vi "InitGalvo.vi"(0 "Galvo-resource in":T4, 1 "No of runs (min.)":i32=1, 2 "ScanControl":T5=[{"Time [s]"=0.0, "action"=enum."Abs", "channel"=enum."SMoveTime", "value (/s)"=0.00144}, {"Time [s]"=0.0, "action"=enum."Abs", "channel"=enum."GalvoX", "value (/s)"=-3.625e-05}, {"Time [s]"=0.0, "action"=enum."Abs", "channel"=enum."GalvoY", "value (/s)"=-4.3125e-05}, {"Time [s]"=0.0, "action"=enum."Abs", "channel"=enum."Galvo3", "value (/s)"=0.0}, {"Time [s]"=0.0, "action"=enum."Abs", "channel"=enum."Image1X", "value (/s)"=0.0}, {"Time [s]"=0.0, "action"=enum."Abs", "channel"=enum."Image1Y", "value (/s)"=0.0}, {"Time [s]"=0.0, "action"=enum."Abs", "channel"=enum."AnalogConfig", "value (/s)"=2.0}, {"Time [s]"=0.0, "action"=enum."LoopStart", "channel"=enum."Loop", "value (/s)"=199.0}, {"Time [s]"=0.0, "action"=enum."Inc", "channel"=enum."GalvoX", "value (/s)"=0.0143229167}, {"Time [s]"=0.0, "action"=enum."Inc", "channel"=enum."GalvoY", "value (/s)"=0.0}, {"Time [s]"=0.0, "action"=enum."Inc", "channel"=enum."Galvo3", "value (/s)"=83333.3333333333}, {"Time [s]"=0.0, "action"=enum."Inc", "channel"=enum."Image1X", "value (/s)"=0.0}, {"Time [s]"=1.2e-05, "action"=enum."Inc", "channel"=enum."Image1X", "value (/s)"=83333.3333333333}, {"Time [s]"=0.0048, "action"=enum."Inc", "channel"=enum."Image1X", "value (/s)"=0.0}, {"Time [s]"=0.0048, "action"=enum."Rel", "channel"=enum."Image1Y", "value (/s)"=1.0}, {"Time [s]"=0.004812, "action"=enum."Abs", "channel"=enum."AnalogConfig", "value (/s)"=3.0}, {"Time [s]"=0.004812, "action"=enum."Inc", "channel"=enum."GalvoX", "value (/s)"=3.5717996675e-05}, {"Time [s]"=0.004812, "action"=enum."Inc", "channel"=enum."GalvoY", "value (/s)"=-2.7275561097e-05}, {"Time [s]"=0.004812, "action"=enum."Inc", "channel"=enum."Galvo3", "value (/s)"=0.0}, {"Time [s]"=0.0, "action"=enum."Abs", "channel"=enum."AnalogConfig", "value (/s)"=2.0}, {"Time [s]"=0.0, "action"=enum."Inc", "channel"=enum."GalvoX", "value (/s)"=-0.0143229167}, {"Time [s]"=0.0, "action"=enum."Inc", "channel"=enum."GalvoY", "value (/s)"=0.0}, {"Time [s]"=0.0, "action"=enum."Inc", "channel"=enum."Galvo3", "value (/s)"=-83333.3333333333}, {"Time [s]"=0.0, "action"=enum."Inc", "channel"=enum."Image1X", "value (/s)"=0.0}, {"Time [s]"=1.2e-05, "action"=enum."Inc", "channel"=enum."Image1X", "value (/s)"=-83333.3333333333}, {"Time [s]"=0.0048, "action"=enum."Inc", "channel"=enum."Image1X", "value (/s)"=0.0}, {"Time [s]"=0.0048, "action"=enum."Rel", "channel"=enum."Image1Y", "value (/s)"=1.0}, {"Time [s]"=0.004812, "action"=enum."Abs", "channel"=enum."AnalogConfig", "value (/s)"=3.0}, {"Time [s]"=0.004812, "action"=enum."Inc", "channel"=enum."GalvoX", "value (/s)"=-3.5717996675e-05}, {"Time [s]"=0.004812, "action"=enum."Inc", "channel"=enum."GalvoY", "value (/s)"=-2.7275561097e-05}, {"Time [s]"=0.004812, "action"=enum."Inc", "channel"=enum."Galvo3", "value (/s)"=0.0}, {"Time [s]"=0.0, "action"=enum."Abs", "channel"=enum."AnalogConfig", "value (/s)"=2.0}, {"Time [s]"=0.0, "action"=enum."LoopEnd", "channel"=enum."Loop", "value (/s)"=0.0}, {"Time [s]"=0.0, "action"=enum."Inc", "channel"=enum."GalvoX", "value (/s)"=0.0143229167}, {"Time [s]"=0.0, "action"=enum."Inc", "channel"=enum."GalvoY", "value (/s)"=0.0}, {"Time [s]"=0.0, "action"=enum."Inc", "channel"=enum."Galvo3", "value (/s)"=83333.3333333333}, {"Time [s]"=0.0, "action"=enum."Inc", "channel"=enum."Image1X", "value (/s)"=0.0}, {"Time [s]"=1.2e-05, "action"=enum."Inc", "channel"=enum."Image1X", "value (/s)"=83333.3333333333}, {"Time [s]"=0.0048, "action"=enum."Inc", "channel"=enum."Image1X", "value (/s)"=0.0}, {"Time [s]"=0.0048, "action"=enum."Rel", "channel"=enum."Image1Y", "value (/s)"=1.0}, {"Time [s]"=0.004812, "action"=enum."Abs", "channel"=enum."AnalogConfig", "value (/s)"=3.0}, {"Time [s]"=0.004812, "action"=enum."Inc", "channel"=enum."GalvoX", "value (/s)"=3.5717996675e-05}, {"Time [s]"=0.004812, "action"=enum."Inc", "channel"=enum."GalvoY", "value (/s)"=-2.7275561097e-05}, {"Time [s]"=0.004812, "action"=enum."Inc", "channel"=enum."Galvo3", "value (/s)"=0.0}, {"Time [s]"=0.0, "action"=enum."Abs", "channel"=enum."AnalogConfig", "value (/s)"=2.0}, {"Time [s]"=0.0, "action"=enum."Inc", "channel"=enum."GalvoX", "value (/s)"=-0.0143229167}, {"Time [s]"=0.0, "action"=enum."Inc", "channel"=enum."GalvoY", "value (/s)"=0.0}, {"Time [s]"=0.0, "action"=enum."Inc", "channel"=enum."Galvo3", "value (/s)"=-83333.3333333333}, {"Time [s]"=0.0, "action"=enum."Inc", "channel"=enum."Image1X", "value (/s)"=0.0}, {"Time [s]"=1.2e-05, "action"=enum."Inc", "channel"=enum."Image1X", "value (/s)"=-83333.3333333333}, {"Time [s]"=0.0048, "action"=enum."Inc", "channel"=enum."GalvoX", "value (/s)"=0.0}, {"Time [s]"=0.0048, "action"=enum."Inc", "channel"=enum."GalvoY", "value (/s)"=0.0}, {"Time [s]"=0.0048, "action"=enum."Inc", "channel"=enum."Galvo3", "value (/s)"=0.0}, {"Time [s]"=0.0048, "action"=enum."Inc", "channel"=enum."Image1X", "value (/s)"=0.0}, {"Time [s]"=0.0048, "action"=enum."Abs", "channel"=enum."AnalogConfig", "value (/s)"=0.0}], 3 "Timing":T1={"AD-clock"=4000000.0, "external ADclock"=TRUE, "Galvocycle"=1e-05, "Bitsize"=1e-07, "AD.start.delay"=0.0, "AddStartTriggerIn"=FALSE, "VoltageRange"={"min Voltage"=-0.1, "max Voltage"=10.0}}, 5 "error in (no error)":errorcluster) -> (6 "Galvo-resource out":T4, 7 "Exact duration/run":dbl, 8 "error out":errorcluster={"status"=TRUE, "code"=-1073807339, "source"="VISA Write in InitGalvo.vi->2PhotonImaging_imaq.vi"})   [LabVIEW 2011]
uses:
  Library/ScanControl/ScanControl.ctl
  Library/ScanControl/ScanControl_Action.ctl
  Library/ScanControl/ScanControl_Channel.ctl
  SIAM/SIAM_command.ctl
  SIAM/SIAM-send.ctl
  <vilib>/DAQmx/write.llb/DAQmx Write (Analog 2D I16 NChan NSamp).vi
  <vilib>/DAQmx/create/channels.llb/DAQmx Create Channel (AO-Voltage-Basic).vi
  <vilib>/DAQmx/configure/timing.llb/DAQmx Timing (Sample Clock).vi
  <vilib>/DAQmx/miscellaneous.llb/DAQmx Fill In Error Info.vi
  National Instruments/LabVIEW 2011/resource/objmgr/daqmx.rc
panel:
  out "Tab Control":enum32{"none", "DSP", "Aout", "SIAM"}(tab)=enum."DSP"
  out "Bytes":i32
  out "FromDSP":string
  out "StringToDSP":string="C\nAV,0,3,-663734\r\nAV,0,4,-789615\r\nAV,0,5,0\r\nAI,0,3,3147\r\nAI,0,4,0\r\nAI,0,5,0\r\nAI,0,3,-3147\r\nAI,0,4,0\r\nAI,0,5,0\r\nAI,0,3,3147\r\nAI,0,4,0\r\nAI,0,5,0\r\nAI,0,3,-3147\r\nAI,0,4,0\r\nAI,0,5,0\r\nAI,0,3,3147\r\nAI,0,4,0\r\nAI,0,5,0\r\nAI,0,3,-3147\r\nAI,0,4,0\r\nAI,0,5,0\r\nAI,0,3,3147\r\nAI,0,4,0\r\nAI,0,5,0\r\nAI,0,3,-3147\r\nAI,0,4,0\r\nAI,0,5,0\r\nAI,0,3,3147\r\nAI,0,4,0\r\nAI,0,5,0\r\nAI,0,3,-3147\r\nAI,0,4,0\r\nAI,0,5,0\r\nAI,0,3,3147\r\nAI,0,4,0\r\nAI,0,5,0\r\nAI,0,3,-3147\r\nAI,0,4,0\r\nAI,0,5,0\r\nAI,0,3,3147\r\nAI,0,4,0\r\nAI,0,5,0\r\nAI,0,3,-3147\r\nAI,0,4,0\r\nAI,0,5,0\r\nAI,0,3,3147\r\nAI,0,4,0\r\nAI,0,5,0\r\nAI,0,3,-3147\r\nAI,0,4,0\r\nAI,0,5,0\r\nAI,0,3,3147\r\nAI,0,4,0\r\nAI,0,5,0\r\nAI,0,3,-3147\r\nAI,0,4,0\r\nAI,0,5,0\r\nAI,0,3,3147\r\nAI,0,4,0\r\nAI,0,5,0\r\nAI,0,3,-3147\r\nAI,0,4,0\r\nAI,0,5,0\r\nAI,0,3,3147\r\nAI,0,4,0\r\nAI,0,5,0\r\nAI,0,3,-3147\r\nAI,0,4,0\r\nAI,0,5,0\r\nAI,0,3,3147\r\nAI,0,4,0\r\nAI,0,5,0\r\nAI,0,3,-3147\r\nAI,0,4,0\r\nAI,0,5,0\r\nAI,0,3,3147\r\nAI,0,4,0\r\nAI,0,5,0\r\nAI,0,3,-3147\r\nAI,0,4,0\r\nAI,0,5,0\r\nAI,0,3,3147\r\nAI,0,4,0\r\nAI,0,5,0\r\nAI,0,3,-3147\r\nAI,0,4,0\r\nAI,0,5,0\r\nAI,0,3,3147\r\nAI,0,4,0\r\nAI,0,5,0\r\nAI,0,3,-3147\r\nAI,0,4,0\r\nAI,0,5,0\r\nAI,0,3,3147\r\nAI,0,4,0\r\nAI,0,5,0\r\nAI,0,3,-3147\r\nAI,0,4,0\r\nAI,0,5,0\r\nAI,0,3,3147\r\nAI,0,4,0\r\nAI,0,5,0\r\nAI,0,3,-3147\r\nAI,0,4,0\r\nAI,0,5,0\r\nAI,0,3,3147\r\nAI,0,4,0\r\nAI,0,5,0\r\nAI,0,3,-3147\r\nAI,0,4,0\r\nAI,0,5,0\r\nAI,0,3,3147\r\nAI,0,4,0\r\nAI,0,5,0\r\nAI,0,3,-3147\r\nAI,0,4,0\r\nAI,0,5,0\r\nAI,0,3,3147\r\nAI,0,4,0\r\nAI,0,5,0\r\nAI,0,3,-3147\r\nAI,0,4,0\r\nAI,0,5,0\r\nAI,0,3,3147\r\nAI,0,4,0\r\nAI,0,5,0\r\nAI,0,3,-3147\r\nAI,0,4,0\r\nAI,0,5,0\r\nAI,0,3,3147\r\nAI,0,4,0\r\nAI,0,5,0\r\nAI,0,3,-3147\r\nAI,0,4,0\r\nAI,0,5,0\r\nAI,0,3,3147\r\nAI,0,4,0\r\nAI,0,5,0\r\nAI,0,3,-3147\r\nAI,0,4,0\r\nAI,0,5,0\r\nAI,0,3,3147\r\nAI,0,4,0\r\nAI,0,5,0\r\nAI,0,3,-3147\r\nAI,0,4,0\r\nAI,0,5,0\r\nAI,0,3,3147\r\nAI,0,4,0\r\nAI,0,5,0\r\nAI,0,3,-3147\r\nAI,0,4,0\r\nAI,0,5,0\r\nAI,0,3,3147\r\nAI,0,4,0\r\nAI,0,5,0\r\nAI,0,3,-3147\r\nAI,0,4,0\r\nAI,0,5,0\r\nAI,0,3,3147\r\nAI,0,4,0\r\nAI,0,5,0\r\nAI,0,3,-3147\r\nAI,0,4,0\r\nAI,0,5,0\r\nAI,0,3,3147\r\nAI,0,4,0\r\nAI,0,5,0\r\nAI,0,3,-3147\r\nAI,0,4,0\r\nAI,0,5,0\r\nAI,0,3,3147\r\nAI,0,4,0\r\nAI,0,5,0\r\nAI,0,3,-3147\r\nAI,0,4,0\r\nAI,0,5,0\r\nAI,0,3,3147\r\nAI,0,4,0\r\nAI,0,5,0\r\nAI,0,3,-3147\r\nAI,0,4,0\r\nAI,0,5,0\r\nAI,0,3,3147\r\nAI,0,4,0\r\nAI,0,5,0\r\nAI,0,3,-3147\r\nAI,0,4,0\r\nAI,0,5,0\r\nAI,0,3,3147\r\nAI,0,4,0\r\nAI,0,5,0\r\nAI,0,3,-3147\r\nAI,0,4,0\r\nAI,0,5,0\r\nAI,0,3,3147\r\nAI,0,4,0\r\nAI,0,5,0\r\nAI,0,3,-3147\r\nAI,0,4,0\r\nAI,0,5,0\r\nAI,0,3,3147\r\nAI,0,4,0\r\nAI,0,5,0\r\nAI,0,3,-3147\r\nAI,0,4,0\r\nAI,0,5,0\r\nAI,0,3,3147\r\nAI,0,4,0\r\nAI,0,5,0\r\nAI,0,3,-3147\r\nAI,0,4,0\r\nAI,0,5,0\r\nAI,0,3,3147\r\nAI,0,4,0\r\nAI,0,5,0\r\nAI,0,3,-3147\r\nAI,0,4,0\r\nAI,0,5,0\r\nAI,0,3,3147\r\nAI,0,4,0\r\nAI,0,5,0\r\nAI,0,3,-3147\r\nAI,0,4,0\r\nAI,0,5,0\r\nAI,0,3,3147\r\nAI,0,4,0\r\nAI,0,5,0\r\nAI,0,3,-3147\r\nAI,0,4,0\r\nAI,0,5,0\r\nAI,0,3,3147\r\nAI,0,4,0\r\nAI,0,5,0\r\nAI,0,3,-3147\r\nAI,0,4,0\r\nAI,0,5,0\r\nAI,0,3,3147\r\nAI,0,4,0\r\nAI,0,5,0\r\nAI,0,3,-3147\r\nAI,0,4,0\r\nAI,0,5,0\r\nAI,0,3,3147\r\nAI,0,4,0\r\nAI,0,5,0\r\nAI,0,3,-3147\r\nAI,0,4,0\r\nAI,0,5,0\r\nAI,0,3,3147\r\nAI,0,4,0\r\nAI,0,5,0\r\nAI,0,3,-3147\r\nAI,0,4,0\r\nAI,0,5,0\r\nAI,0,3,3147\r\nAI,0,4,0\r\nAI,0,5,0\r\nAI,0,3,-3147\r\nAI,0,4,0\r\nAI,0,5,0\r\nAI,0,3,3147\r\nAI,0,4,0\r\nAI,0,5,0\r\nAI,0,3,-3147\r\nAI,0,4,0\r\nAI,0,5,0\r\nAI,0,3,3147\r\nAI,0,4,0\r\nAI,0,5,0\r\nAI,0,3,-3147\r\nAI,0,4,0\r\nAI,0,5,0\r\nAI,0,3,3147\r\nAI,0,4,0\r\nAI,0,5,0\r\nAI,0,3,-3147\r\nAI,0,4,0\r\nAI,0,5,0\r\nAI,0,3,3147\r\nAI,0,4,0\r\nAI,0,5,0\r\nAI,0,3,-3147\r\nAI,0,4,0\r\nAI,0,5,0\r\nAI,0,3,3147\r\nAI,0,4,0\r\nAI,0,5,0\r\nAI,0,3,-3147\r\nAI,0,4,0\r\nAI,0,5,0\r\nAI,0,3,3147\r\nAI,0,4,0\r\nAI,0,5,0\r\nAI,0,3,-3147\r\nAI,0,4,0\r\nAI,0,5,0\r\nAI,0,3,3147\r\nAI,0,4,0\r\nAI,0,5,0\r\nAI,0,3,-3147\r\nAI,0,4,0\r\nAI,0,5,0\r\nAI,0,3,3147\r\nAI,0,4,0\r\nAI,0,5,0\r\nAI,0,3,-3147\r\nAI,0,4,0\r\nAI,0,5,0\r\nAI,0,3,3147\r\nAI,0,4,0\r\nAI,0,5,0\r\nAI,0,3,-3147\r\nAI,0,4,0\r\nAI,0,5,0\r\nAI,0,3,3147\r\nAI,0,4,0\r\nAI,0,5,0\r\nAI,0,3,-3147\r\nAI,0,4,0\r\nAI,0,5,0\r\nAI,0,3,3147\r\nAI,0,4,0\r\nAI,0,5,0\r\nAI,0,3,-3147\r\nAI,0,4,0\r\nAI,0,5,0\r\nAI,0,3,3147\r\nAI,0,4,0\r\nAI,0,5,0\r\nAI,0,3,-3147\r\nAI,0,4,0\r\nAI,0,5,0\r\nAI,0,3,3147\r\nAI,0,4,0\r\nAI,0,5,0\r\nAI,0,3,-3147\r\nAI,0,4,0\r\nAI,0,5,0\r\nAI,0,3,3147\r\nAI,0,4,0\r\nAI,0,5,0\r\nAI,0,3,-3147\r\nAI,0,4,0\r\nAI,0,5,0\r\nAI,0,3,3147\r\nAI,0,4,0\r\nAI,0,5,0\r\nAI,0,3,-3147\r\nAI,0,4,0\r\nAI,0,5,0\r\nAI,0,3,3147\r\nAI,0,4,0\r\nAI,0,5,0\r\nAI,0,3,-3147\r\nAI,0,4,0\r\nAI,0,5,0\r\nAI,0,3,3147\r\nAI,0,4,0\r\nAI,0,5,0\r\nAI,0,3,-3147\r\nAI,0,4,0\r\nAI,0,5,0\r\nAI,0,3,3147\r\nAI,0,4,0\r\nAI,0,5,0\r\nAI,0,3,-3147\r\nAI,0,4,0\r\nAI,0,5,0\r\nAI,0,3,3147\r\nAI,0,4,0\r\nAI,0,5,0\r\nAI,0,3,-3147\r\nAI,0,4,0\r\nAI,0,5,0\r\nAI,0,3,3147\r\nAI,0,4,0\r\nAI,0,5,0\r\nAI,0,3,-3147\r\nAI,0,4,0\r\nAI,0,5,0\r\nAI,0,3,3147\r\nAI,0,4,0\r\nAI,0,5,0\r\nAI,0,3,-3147\r\nAI,0,4,0\r\nAI,0,5,0\r\nAI,0,3,3147\r\nAI,0,4,0\r\nAI,0,5,0\r\nAI,0,3,-3147\r\nAI,0,4,0\r\nAI,0,5,0\r\nAI,0,3,3147\r\nAI,0,4,0\r\nAI,0,5,0\r\nAI,0,3,-3147\r\nAI,0,4,0\r\nAI,0,5,0\r\nAI,0,3,3147\r\nAI,0,4,0\r\nAI,0,5,0\r\nAI,0,3,-3147\r\nAI,0,4,0\r\nAI,0,5,0\r\nAI,0,3,3147\r\nAI,0,4,0\r\nAI,0,5,0\r\nAI,0,3,-3147\r\nAI,0,4,0\r\nAI,0,5,0\r\nAI,0,3,3147\r\nAI,0,4,0\r\nAI,0,5,0\r\nAI,0,3,-3147\r\nAI,0,4,0\r\nAI,0,5,0\r\nAI,0,3,3147\r\nAI,0,4,0\r\nAI,0,5,0\r\nAI,0,3,-3147\r\nAI,0,4,0\r\nAI,0,5,0\r\nAI,0,3,3147\r\nAI,0,4,0\r\nAI,0,5,0\r\nAI,0,3,-3147\r\nAI,0,4,0\r\nAI,0,5,0\r\nAI,0,3,3147\r\nAI,0,4,0\r\nAI,0,5,0\r\nAI,0,3,-3147\r\nAI,0,4,0\r\nAI,0,5,0\r\nAI,0,3,3147\r\nAI,0,4,0\r\nAI,0,5,0\r\nAI,0,3,-3147\r\nAI,0,4,0\r\nAI,0,5,0\r\nAI,0,3,3147\r\nAI,0,4,0\r\nAI,0,5,0\r\nAI,0,3,-3147\r\nAI,0,4,0\r\nAI,0,5,0\r\nAI,0,3,3147\r\nAI,0,4,0\r\nAI,0,5,0\r\nAI,0,3,-3147\r\nAI,0,4,0\r\nAI,0,5,0\r\nAI,0,3,3147\r\nAI,0,4,0\r\nAI,0,5,0\r\nAI,0,3,-3147\r\nAI,0,4,0\r\nAI,0,5,0\r\nAI,0,3,3147\r\nAI,0,4,0\r\nAI,0,5,0\r\nAI,0,3,-3147\r\nAI,0,4,0\r\nAI,0,5,0\r\nAI,0,3,3147\r\nAI,0,4,0\r\nAI,0,5,0\r\nAI,0,3,-3147\r\nAI,0,4,0\r\nAI,0,5,0\r\nAI,0,3,3147\r\nAI,0,4,0\r\nAI,0,5,0\r\nAI,0,3,-3147\r\nAI,0,4,0\r\nAI,0,5,0\r\nAI,0,3,3147\r\nAI,0,4,0\r\nAI,0,5,0\r\nAI,0,3,-3147\r\nAI,0,4,0\r\nAI,0,5,0\r\nAI,0,3,3147\r\nAI,0,4,0\r\nAI,0,5,0\r\nAI,0,3,-3147\r\nAI,0,4,0\r\nAI,0,5,0\r\nAI,0,3,3147\r\nAI,0,4,0\r\nAI,0,5,0\r\nAI,0,3,-3147\r\nAI,0,4,0\r\nAI,0,5,0\r\nAI,0,3,3147\r\nAI,0,4,0\r\nAI,0,5,0\r\nAI,0,3,-3147\r\nAI,0,4,0\r\nAI,0,5,0\r\nAI,0,3,3147\r\nAI,0,4,0\r\nAI,0,5,0\r\nAI,0,3,-3147\r\nAI,0,4,0\r\nAI,0,5,0\r\nAI,0,3,3147\r\nAI,0,4,0\r\nAI,0,5,0\r\nAI,0,3,-3147\r\nAI,0,4,0\r\nAI,0,5,0\r\nAI,0,3,3147\r\nAI,0,4,0\r\nAI,0,5,0\r\nAI,0,3,-3147\r\nAI,0,4,0\r\nAI,0,5,0\r\nAI,0,3,3147\r\nAI,0,4,0\r\nAI,0,5,0\r\nAI,0,3,-3147\r\nAI,0,4,0\r\nAI,0,5,0\r\nAI,0,3,3147\r\nAI,0,4,0\r\nAI,0,5,0\r\nAI,0,3,-3147\r\nAI,0,4,0\r\nAI,0,5,0\r\nAI,0,3,3147\r\nAI,0,4,0\r\nAI,0,5,0\r\nAI,0,3,-3147\r\nAI,0,4,0\r\nAI,0,5,0\r\nAI,0,3,3147\r\nAI,0,4,0\r\nAI,0,5,0\r\nAI,0,3,-3147\r\nAI,0,4,0\r\nAI,0,5,0\r\nAI,0,3,3147\r\nAI,0,4,0\r\nAI,0,5,0\r\nAI,0,3,-3147\r\nAI,0,4,0\r\nAI,0,5,0\r\nAI,0,3,3147\r\nAI,0,4,0\r\nAI,0,5,0\r\nAI,0,3,-3147\r\nAI,0,4,0\r\nAI,0,5,0\r\nAI,0,3,3147\r\nAI,0,4,0\r\nAI,0,5,0\r\nAI,0,3,-3147\r\nAI,0,4,0\r\nAI,0,5,0\r\nAI,0,3,3147\r\nAI,0,4,0\r\nAI,0,5,0\r\nAI,0,3,-3147\r\nAI,0,4,0\r\nAI,0,5,0\r\nAI,0,3,3147\r\nAI,0,4,0\r\nAI,0,5,0\r\nAI,0,3,-3147\r\nAI,0,4,0\r\nAI,0,5,0\r\nAI,0,3,3147\r\nAI,0,4,0\r\nAI,0,5,0\r\nAI,0,3,-3147\r\nAI,0,4,0\r\nAI,0,5,0\r\nAI,0,3,3147\r\nAI,0,4,0\r\nAI,0,5,0\r\nAI,0,3,-3147\r\nAI,0,4,0\r\nAI,0,5,0\r\nAI,0,3,3147\r\nAI,0,4,0\r\nAI,0,5,0\r\nAI,0,3,-3147\r\nAI,0,4,0\r\nAI,0,5,0\r\nAI,0,3,3147\r\nAI,0,4,0\r\nAI,0,5,0\r\nAI,0,3,-3147\r\nAI,0,4,0\r\nAI,0,5,0\r\nAI,0,3,3147\r\nAI,0,4,0\r\nAI,0,5,0\r\nAI,0,3,-3147\r\nAI,0,4,0\r\nAI,0,5,0\r\nAI,0,3,3147\r\nAI,0,4,0\r\nAI,0,5,0\r\nAI,0,3,-3147\r\nAI,0,4,0\r\nAI,0,5,0\r\nAI,0,3,3147\r\nAI,0,4,0\r\nAI,0,5,0\r\nAI,0,3,-3147\r\nAI,0,4,0\r\nAI,0,5,0\r\nAI,0,3,3147\r\nAI,0,4,0\r\nAI,0,5,0\r\nAI,0,3,-3147\r\nAI,0,4,0\r\nAI,0,5,0\r\nAI,0,3,3147\r\nAI,0,4,0\r\nAI,0,5,0\r\nAI,0,3,-3147\r\nAI,0,4,0\r\nAI,0,5,0\r\nAI,0,3,3147\r\nAI,0,4,0\r\nAI,0,5,0\r\nAI,0,3,-3147\r\nAI,0,4,0\r\nAI,0,5,0\r\nAI,0,3,3147\r\nAI,0,4,0\r\nAI,0,5,0\r\nAI,0,3,-3147\r\nAI,0,4,0\r\nAI,0,5,0\r\nAI,0,3,3147\r\nAI,0,4,0\r\nAI,0,5,0\r\nAI,0,3,-3147\r\nAI,0,4,0\r\nAI,0,5,0\r\nAI,0,3,3147\r\nAI,0,4,0\r\nAI,0,5,0\r\nAI,0,3,-3147\r\nAI,0,4,0\r\nAI,0,5,0\r\nAI,0,3,3147\r\nAI,0,4,0\r\nAI,0,5,0\r\nAI,0,3,-3147\r\nAI,0,4,0\r\nAI,0,5,0\r\nAI,0,3,3147\r\nAI,0,4,0\r\nAI,0,5,0\r\nAI,0,3,-3147\r\nAI,0,4,0\r\nAI,0,5,0\r\nAI,0,3,3147\r\nAI,0,4,0\r\nAI,0,5,0\r\nAI,0,3,-3147\r\nAI,0,4,0\r\nAI,0,5,0\r\nAI,0,3,3147\r\nAI,0,4,0\r\nAI,0,5,0\r\nAI,0,3,-3147\r\nAI,0,4,0\r\nAI,0,5,0\r\nAI,0,3,3147\r\nAI,0,4,0\r\nAI,0,5,0\r\nAI,0,3,-3147\r\nAI,0,4,0\r\nAI,0,5,0\r\nAI,0,3,3147\r\nAI,0,4,0\r\nAI,0,5,0\r\nAI,0,3,-3147\r\nAI,0,4,0\r\nAI,0,5,0\r\nAI,0,3,3147\r\nAI,0,4,0\r\nAI,0,5,0\r\nAI,0,3,-3147\r\nAI,0,4,0\r\nAI,0,5,0\r\nAI,0,3,3147\r\nAI,0,4,0\r\nAI,0,5,0\r\nAI,0,3,-3147\r\nAI,0,4,0\r\nAI,0,5,0\r\nAI,0,3,3147\r\nAI,0,4,0\r\nAI,0,5,0\r\nAI,0,3,-3147\r\nAI,0,4,0\r\nAI,0,5,0\r\nAI,0,3,3147\r\nAI,0,4,0\r\nAI,0,5,0\r\nAI,0,3,-3147\r\nAI,0,4,0\r\nAI,0,5,0\r\nAI,0,3,3147\r\nAI,0,4,0\r\nAI,0,5,0\r\nAI,0,3,-3147\r\nAI,0,4,0\r\nAI,0,5,0\r\nAI,0,3,3147\r\nAI,0,4,0\r\nAI,0,5,0\r\nAI,0,3,-3147\r\nAI,0,4,0\r\nAI,0,5,0\r\nAI,0,3,3147\r\nAI,0,4,0\r\nAI,0,5,0\r\nAI,0,3,-3147\r\nAI,0,4,0\r\nAI,0,5,0\r\nAI,0,3,3147\r\nAI,0,4,0\r\nAI,0,5,0\r\nAI,0,3,-3147\r\nAI,0,4,0\r\nAI,0,5,0\r\nAI,0,3,3147\r\nAI,0,4,0\r\nAI,0,5,0\r\nAI,0,3,-3147\r\nAI,0,4,0\r\nAI,0,5,0\r\nAI,0,3,3147\r\nAI,0,4,0\r\nAI,0,5,0\r\nAI,0,3,-3147\r\nAI,0,4,0\r\nAI,0,5,0\r\nAI,0,3,3147\r\nAI,0,4,0\r\nAI,0,5,0\r\nAI,0,3,-3147\r\nAI,0,4,0\r\nAI,0,5,0\r\nAI,0,3,3147\r\nAI,0,4,0\r\nAI,0,5,0\r\nAI,0,3,-3147\r\nAI,0,4,0\r\nAI,0,5,0\r\nAI,0,3,3147\r\nAI,0,4,0\r\nAI,0,5,0\r\nAI,0,3,-3147\r\nAI,0,4,0\r\nAI,0,5,0\r\nAI,0,3,3147\r\nAI,0,4,0\r\nAI,0,5,0\r\nAI,0,3,-3147\r\nAI,0,4,0\r\nAI,0,5,0\r\nAI,0,3,3147\r\nAI,0,4,0\r\nAI,0,5,0\r\nAI,0,3,-3147\r\nAI,0,4,0\r\nAI,0,5,0\r\nAI,0,3,3147\r\nAI,0,4,0\r\nAI,0,5,0\r\nAI,0,3,-3147\r\nAI,0,4,0\r\nAI,0,5,0\r\nAI,0,3,3147\r\nAI,0,4,0\r\nAI,0,5,0\r\nAI,0,3,-3147\r\nAI,0,4,0\r\nAI,0,5,0\r\nAI,0,3,3147\r\nAI,0,4,0\r\nAI,0,5,0\r\nAI,0,3,-3147\r\nAI,0,4,0\r\nAI,0,5,0\r\nAI,0,3,3147\r\nAI,0,4,0\r\nAI,0,5,0\r\nAI,0,3,-3147\r\nAI,0,4,0\r\nAI,0,5,0\r\nAI,0,3,3147\r\nAI,0,4,0\r\nAI,0,5,0\r\nAI,0,3,-3147\r\nAI,0,4,0\r\nAI,0,5,0\r\nAI,0,3,3147\r\nAI,0,4,0\r\nAI,0,5,0\r\nAI,0,3,-3147\r\nAI,0,4,0\r\nAI,0,5,0\r\nAI,0,3,3147\r\nAI,0,4,0\r\nAI,0,5,0\r\nAI,0,3,-3147\r\nAI,0,4,0\r\nAI,0,5,0\r\nAI,0,3,3147\r\nAI,0,4,0\r\nAI,0,5,0\r\nAI,0,3,-3147\r\nAI,0,4,0\r\nAI,0,5,0\r\nAI,0,3,3147\r\nAI,0,4,0\r\nAI,0,5,0\r\nAI,0,3,-3147\r\nAI,0,4,0\r\nAI,0,5,0\r\nAI,0,3,3147\r\nAI,0,4,0\r\nAI,0,5,0\r\nAI,0,3,-3147\r\nAI,0,4,0\r\nAI,0,5,0\r\nAI,0,3,3147\r\nAI,0,4,0\r\nAI,0,5,0\r\nAI,0,3,-3147\r\nAI,0,4,0\r\nAI,0,5,0\r\nAI,0,3,3147\r\nAI,0,4,0\r\nAI,0,5,0\r\nAI,0,3,-3147\r\nAI,0,4,0\r\nAI,0,5,0\r\nAI,0,3,3147\r\nAI,0,4,0\r\nAI,0,5,0\r\nAI,0,3,-3147\r\nAI,0,4,0\r\nAI,0,5,0\r\nAI,0,3,3147\r\nAI,0,4,0\r\nAI,0,5,0\r\nAI,0,3,-3147\r\nAI,0,4,0\r\nAI,0,5,0\r\nAI,0,3,3147\r\nAI,0,4,0\r\nAI,0,5,0\r\nAI,0,3,-3147\r\nAI,0,4,0\r\nAI,0,5,0\r\nAI,0,3,3147\r\nAI,0,4,0\r\nAI,0,5,0\r\nAI,0,3,-3147\r\nAI,0,4,0\r\nAI,0,5,0\r\nAI,0,3,3147\r\nAI,0,4,0\r\nAI,0,5,0\r\nAI,0,3,-3147\r\nAI,0,4,0\r\nAI,0,5,0\r\nAI,0,3,3147\r\nAI,0,4,0\r\nAI,0,5,0\r\nAI,0,3,-3147\r\nAI,0,4,0\r\nAI,0,5,0\r\nAI,0,3,3147\r\nAI,0,4,0\r\nAI,0,5,0\r\nAI,0,3,-3147\r\nAI,0,4,0\r\nAI,0,5,0\r\nAI,0,3,3147\r\nAI,0,4,0\r\nAI,0,5,0\r\nAI,0,3,-3147\r\nAI,0,4,0\r\nAI,0,5,0\r\nAI,0,3,3147\r\nAI,0,4,0\r\nAI,0,5,0\r\nAI,0,3,-3147\r\nAI,0,4,0\r\nAI,0,5,0\r\nAI,0,3,3147\r\nAI,0,4,0\r\nAI,0,5,0\r\nAI,0,3,-3147\r\nAI,0,4,0\r\nAI,0,5,0\r\nAI,0,3,3147\r\nAI,0,4,0\r\nAI,0,5,0\r\nAI,0,3,-3147\r\nAI,0,4,0\r\nAI,0,5,0\r\nAI,0,3,3147\r\nAI,0,4,0\r\nAI,0,5,0\r\nAI,0,3,-3147\r\nAI,0,4,0\r\nAI,0,5,0\r\nAI,0,3,3147\r\nAI,0,4,0\r\nAI,0,5,0\r\nAI,0,3,-3147\r\nAI,0,4,0\r\nAI,0,5,0\r\nAI,0,3,3147\r\nAI,0,4,0\r\nAI,0,5,0\r\nAI,0,3,-3147\r\nAI,0,4,0\r\nAI,0,5,0\r\nAI,0,3,3147\r\nAI,0,4,0\r\nAI,0,5,0\r\nAI,0,3,-3147\r\nAI,0,4,0\r\nAI,0,5,0\r\nAI,0,3,3147\r\nAI,0,4,0\r\nAI,0,5,0\r\nAI,0,3,-3147\r\nAI,0,4,0\r\nAI,0,5,0\r\nAI,0,3,3147\r\nAI,0,4,0\r\nAI,0,5,0\r\nAI,0,3,-3147\r\nAI,0,4,0\r\nAI,0,5,0\r\nAI,0,3,3147\r\nAI,0,4,0\r\nAI,0,5,0\r\nAI,0,3,-3147\r\nAI,0,4,0\r\nAI,0,5,0\r\nAI,0,3,3147\r\nAI,0,4,0\r\nAI,0,5,0\r\nAI,0,3,-3147\r\nAI,0,4,0\r\nAI,0,5,0\r\nAI,0,3,3147\r\nAI,0,4,0\r\nAI,0,5,0\r\nAI,0,3,-3147\r\nAI,0,4,0\r\nAI,0,5,0\r\nAI,0,3,3147\r\nAI,0,4,0\r\nAI,0,5,0\r\nAI,0,3,-3147\r\nAI,0,4,0\r\nAI,0,5,0\r\nAI,0,3,3147\r\nAI,0,4,0\r\nAI,0,5,0\r\nAI,0,3,-3147\r\nAI,0,4,0\r\nAI,0,5,0\r\nAI,0,3,3147\r\nAI,0,4,0\r\nAI,0,5,0\r\nAI,0,3,-3147\r\nAI,0,4,0\r\nAI,0,5,0\r\nAI,0,3,3147\r\nAI,0,4,0\r\nAI,0,5,0\r\nAI,0,3,-3147\r\nAI,0,4,0\r\nAI,0,5,0\r\nAI,0,3,3147\r\nAI,0,4,0\r\nAI,0,5,0\r\nAI,0,3,-3147\r\nAI,0,4,0\r\nAI,0,5,0\r\nAI,0,3,3147\r\nAI,0,4,0\r\nAI,0,5,0\r\nAI,0,3,-3147\r\nAI,0,4,0\r\nAI,0,5,0\r\nAI,0,3,3147\r\nAI,0,4,0\r\nAI,0,5,0\r\nAI,0,3,-3147\r\nAI,0,4,0\r\nAI,0,5,0\r\nAI,0,3,3147\r\nAI,0,4,0\r\nAI,0,5,0\r\nAI,0,3,-3147\r\nAI,0,4,0\r\nAI,0,5,0\r\nAI,0,3,3147\r\nAI,0,4,0\r\nAI,0,5,0\r\nAI,0,3,-3147\r\nAI,0,4,0\r\nAI,0,5,0\r\nAI,0,3,3147\r\nAI,0,4,0\r\nAI,0,5,0\r\nAI,0,3,-3147\r\nAI,0,4,0\r\nAI,0,5,0\r\nAI,0,3,3147\r\nAI,0,4,0\r\nAI,0,5,0\r\nAI,0,3,-3147\r\nAI,0,4,0\r\nAI,0,5,0\r\nAI,0,3,3147\r\nAI,0,4,0\r\nAI,0,5,0\r\nAI,0,3,-3147\r\nAI,0,4,0\r\nAI,0,5,0\r\nAI,0,3,3147\r\nAI,0,4,0\r\nAI,0,5,0\r\nAI,0,3,-3147\r\nAI,0,4,0\r\nAI,0,5,0\r\nAI,0,3,3147\r\nAI,0,4,0\r\nAI,0,5,0\r\nAI,0,3,-3147\r\nAI,0,4,0\r\nAI,0,5,0\r\nAI,0,3,3147\r\nAI,0,4,0\r\nAI,0,5,0\r\nAI,0,3,-3147\r\nAI,0,4,0\r\nAI,0,5,0\r\nAI,0,3,3147\r\nAI,0,4,0\r\nAI,0,5,0\r\nAI,0,3,-3147\r\nAI,0,4,0\r\nAI,0,5,0\r\nAI,0,3,3147\r\nAI,0,4,0\r\nAI,0,5,0\r\nAI,0,3,-3147\r\nAI,0,4,0\r\nAI,0,5,0\r\nAI,0,3,3147\r\nAI,0,4,0\r\nAI,0,5,0\r\nAI,0,3,-3147\r\nAI,0,4,0\r\nAI,0,5,0\r\nAI,0,3,3147\r\nAI,0,4,0\r\nAI,0,5,0\r\nAI,0,3,-3147\r\nAI,0,4,0\r\nAI,0,5,0\r\nAI,0,3,3147\r\nAI,0,4,0\r\nAI,0,5,0\r\nAI,0,3,-3147\r\nAI,0,4,0\r\nAI,0,5,0\r\nAI,0,3,3147\r\nAI,0,4,0\r\nAI,0,5,0\r\nAI,0,3,-3147\r\nAI,0,4,0\r\nAI,0,5,0\r\nAI,0,3,3147\r\nAI,0,4,0\r\nAI,0,5,0\r\nAI,0,3,-3147\r\nAI,0,4,0\r\nAI,0,5,0\r\nAI,0,3,3147\r\nAI,0,4,0\r\nAI,0,5,0\r\nAI,0,3,-3147\r\nAI,0,4,0\r\nAI,0,5,0\r\nAI,0,3,3147\r\nAI,0,4,0\r\nAI,0,5,0\r\nAI,0,3,-3147\r\nAI,0,4,0\r\nAI,0,5,0\r\nAI,0,3,3147\r\nAI,0,4,0\r\nAI,0,5,0\r\nAI,0,3,-3147\r\nAI,0,4,0\r\nAI,0,5,0\r\nAI,0,3,3147\r\nAI,0,4,0\r\nAI,0,5,0\r\nAI,0,3,-3147\r\nAI,0,4,0\r\nAI,0,5,0\r\nAI,0,3,3147\r\nAI,0,4,0\r\nAI,0,5,0\r\nAI,0,3,-3147\r\nAI,0,4,0\r\nAI,0,5,0\r\nAI,0,3,3147\r\nAI,0,4,0\r\nAI,0,5,0\r\nAI,0,3,-3147\r\nAI,0,4,0\r\nAI,0,5,0\r\nAI,0,3,3147\r\nAI,0,4,0\r\nAI,0,5,0\r\nAI,0,3,-3147\r\nAI,0,4,0\r\nAI,0,5,0\r\nAI,0,3,3147\r\nAI,0,4,0\r\nAI,0,5,0\r\nAI,0,3,-3147\r\nAI,0,4,0\r\nAI,0,5,0\r\nAI,0,3,3147\r\nAI,0,4,0\r\nAI,0,5,0\r\nAI,0,3,-3147\r\nAI,0,4,0\r\nAI,0,5,0\r\nAI,0,3,3147\r\nAI,0,4,0\r\nAI,0,5,0\r\nAI,0,3,-3147\r\nAI,0,4,0\r\nAI,0,5,0\r\nAI,0,3,3147\r\nAI,0,4,0\r\nAI,0,5,0\r\nAI,0,3,-3147\r\nAI,0,4,0\r\nAI,0,5,0\r\nAI,0,3,3147\r\nAI,0,4,0\r\nAI,0,5,0\r\nAI,0,3,-3147\r\nAI,0,4,0\r\nAI,0,5,0\r\nAI,0,3,3147\r\nAI,0,4,0\r\nAI,0,5,0\r\nAI,0,3,-3147\r\nAI,0,4,0\r\nAI,0,5,0\r\nAI,0,3,3147\r\nAI,0,4,0\r\nAI,0,5,0\r\nAI,0,3,-3147\r\nAI,0,4,0\r\nAI,0,5,0\r\nAI,0,3,3147\r\nAI,0,4,0\r\nAI,0,5,0\r\nAI,0,3,-3147\r\nAI,0,4,0\r\nAI,0,5,0\r\nAI,0,3,3147\r\nAI,0,4,0\r\nAI,0,5,0\r\nAI,0,3,-3147\r\nAI,0,4,0\r\nAI,0,5,0\r\nAI,0,3,3147\r\nAI,0,4,0\r\nAI,0,5,0\r\nAI,0,3,-3147\r\nAI,0,4,0\r\nAI,0,5,0\r\nAV,120,1,2\r\nAV,120,1,2\r\nAV,120,1,2\r\nAV,120,1,2\r\nAV,120,1,2\r\nAV,120,1,2\r\nAV,120,1,2\r\nAV,120,1,2\r\nAV,120,1,2\r\nAV,120,1,2\r\nAV,120,1,2\r\nAV,120,1,2\r\nAV,120,1,2\r\nAV,120,1,2\r\nAV,120,1,2\r\nAV,120,1,2\r\nAV,120,1,2\r\nAV,120,1,2\r\nAV,120,1,2\r\nAV,120,1,2\r\nAV,120,1,2\r\nAV,120,1,2\r\nAV,120,1,2\r\nAV,120,1,2\r\nAV,120,1,2\r\nAV,120,1,2\r\nAV,120,1,2\r\nAV,120,1,2\r\nAV,120,1,2\r\nAV,120,1,2\r\nAV,120,1,2\r\nAV,120,1,2\r\nAV,120,1,2\r\nAV,120,1,2\r\nAV,120,1,2\r\nAV,120,1,2\r\nAV,120,1,2\r\nAV,120,1,2\r\nAV,120,1,2\r\nAV,120,1,2\r\nAV,120,1,2\r\nAV,120,1,2\r\nAV,120,1,2\r\nAV,120,1,2\r\nAV,120,1,2\r\nAV,120,1,2\r\nAV,120,1,2\r\nAV,120,1,2\r\nAV,120,1,2\r\nAV,120,1,2\r\nAV,120,1,2\r\nAV,120,1,2\r\nAV,120,1,2\r\nAV,120,1,2\r\nAV,120,1,2\r\nAV,120,1,2\r\nAV,120,1,2\r\nAV,120,1,2\r\nAV,120,1,2\r\nAV,120,1,2\r\nAV,120,1,2\r\nAV,120,1,2\r\nAV,120,1,2\r\nAV,120,1,2\r\nAV,120,1,2\r\nAV,120,1,2\r\nAV,120,1,2\r\nAV,120,1,2\r\nAV,120,1,2\r\nAV,120,1,2\r\nAV,120,1,2\r\nAV,120,1,2\r\nAV,120,1,2\r\nAV,120,1,2\r\nAV,120,1,2\r\nAV,120,1,2\r\nAV,120,1,2\r\nAV,120,1,2\r\nAV,120,1,2\r\nAV,120,1,2\r\nAV,120,1,2\r\nAV,120,1,2\r\nAV,120,1,2\r\nAV,120,1,2\r\nAV,120,1,2\r\nAV,120,1,2\r\nAV,120,1,2\r\nAV,120,1,2\r\nAV,120,1,2\r\nAV,120,1,2\r\nAV,120,1,2\r\nAV,120,1,2\r\nAV,120,1,2\r\nAV,120,1,2\r\nAV,120,1,2\r\nAV,120,1,2\r\nAV,120,1,2\r\nAV,120,1,2\r\nAV,120,1,2\r\nAV,120,1,2\r\nAV,120,1,2\r\nAV,120,1,2\r\nAV,120,1,2\r\nAV,120,1,2\r\nAV,120,1,2\r\nAV,120,1,2\r\nAV,120,1,2\r\nAV,120,1,2\r\nAV,120,1,2\r\nAV,120,1,2\r\nAV,120,1,2\r\nAV,120,1,2\r\nAV,120,1,2\r\nAV,120,1,2\r\nAV,120,1,2\r\nAV,120,1,2\r\nAV,120,1,2\r\nAV,120,1,2\r\nAV,120,1,2\r\nAV,120,1,2\r\nAV,120,1,2\r\nAV,120,1,2\r\nAV,120,1,2\r\nAV,120,1,2\r\nAV,120,1,2\r\nAV,120,1,2\r\nAV,120,1,2\r\nAV,120,1,2\r\nAV,120,1,2\r\nAV,120,1,2\r\nAV,120,1,2\r\nAV,120,1,2\r\nAV,120,1,2\r\nAV,120,1,2\r\nAV,120,1,2\r\nAV,120,1,2\r\nAV,120,1,2\r\nAV,120,1,2\r\nAV,120,1,2\r\nAV,120,1,2\r\nAV,120,1,2\r\nAV,120,1,2\r\nAV,120,1,2\r\nAV,120,1,2\r\nAV,120,1,2\r\nAV,120,1,2\r\nAV,120,1,2\r\nAV,120,1,2\r\nAV,120,1,2\r\nAV,120,1,2\r\nAV,120,1,2\r\nAV,120,1,2\r\nAV,120,1,2\r\nAV,120,1,2\r\nAV,120,1,2\r\nAV,120,1,2\r\nAV,120,1,2\r\nAV,120,1,2\r\nAV,120,1,2\r\nAV,120,1,2\r\nAV,120,1,2\r\nAV,120,1,2\r\nAV,120,1,2\r\nAV,120,1,2\r\nAV,120,1,2\r\nAV,120,1,2\r\nAV,120,1,2\r\nAV,120,1,2\r\nAV,120,1,2\r\nAV,120,1,2\r\nAV,120,1,2\r\nAV,120,1,2\r\nAV,120,1,2\r\nAV,120,1,2\r\nAV,120,1,2\r\nAV,120,1,2\r\nAV,120,1,2\r\nAV,120,1,2\r\nAV,120,1,2\r\nAV,120,1,2\r\nAV,120,1,2\r\nAV,120,1,2\r\nAV,120,1,2\r\nAV,120,1,2\r\nAV,120,1,2\r\nAV,120,1,2\r\nAV,120,1,2\r\nAV,120,1,2\r\nAV,120,1,2\r\nAV,120,1,2\r\nAV,120,1,2\r\nAV,120,1,2\r\nAV,120,1,2\r\nAV,120,1,2\r\nAV,120,1,2\r\nAV,120,1,2\r\nAV,120,1,2\r\nAV,120,1,2\r\nAV,120,1,2\r\nAV,120,1,2\r\nAV,120,1,2\r\nAV,120,1,2\r\nAV,120,1,2\r\nAV,120,1,2\r\nAV,120,1,2\r\nAV,120,1,2\r\nAV,120,1,2\r\nAV,120,1,2\r\nAV,120,1,2\r\nAV,120,1,2\r\nAV,120,1,2\r\nAV,120,1,2\r\nAV,120,1,2\r\nAV,120,1,2\r\nAV,120,1,2\r\nAV,120,1,2\r\nAV,120,1,2\r\nAV,120,1,2\r\nAV,120,1,2\r\nAV,120,1,2\r\nAV,120,1,2\r\nAV,120,1,2\r\nAV,120,1,2\r\nAV,120,1,2\r\nAV,120,1,2\r\nAV,120,1,2\r\nAV,120,1,2\r\nAV,120,1,2\r\nAV,120,1,2\r\nAV,120,1,2\r\nAV,120,1,2\r\nAV,120,1,2\r\nAV,120,1,2\r\nAV,120,1,2\r\nAV,120,1,2\r\nAV,120,1,2\r\nAV,120,1,2\r\nAV,120,1,2\r\nAV,120,1,2\r\nAV,120,1,2\r\nAV,120,1,2\r\nAV,120,1,2\r\nAV,120,1,2\r\nAV,120,1,2\r\nAV,120,1,2\r\nAV,120,1,2\r\nAV,120,1,2\r\nAV,120,1,2\r\nAV,120,1,2\r\nAV,120,1,2\r\nAV,120,1,2\r\nAV,120,1,2\r\nAV,120,1,2\r\nAV,120,1,2\r\nAV,120,1,2\r\nAV,120,1,2\r\nAV,120,1,2\r\nAV,120,1,2\r\nAV,120,1,2\r\nAV,120,1,2\r\nAV,120,1,2\r\nAV,120,1,2\r\nAV,120,1,2\r\nAV,120,1,2\r\nAV,120,1,2\r\nAV,120,1,2\r\nAV,120,1,2\r\nAV,120,1,2\r\nAV,120,1,2\r\nAV,120,1,2\r\nAV,120,1,2\r\nAV,120,1,2\r\nAV,120,1,2\r\nAV,120,1,2\r\nAV,120,1,2\r\nAV,120,1,2\r\nAV,120,1,2\r\nAV,120,1,2\r\nAV,120,1,2\r\nAV,120,1,2\r\nAV,120,1,2\r\nAV,120,1,2\r\nAV,120,1,2\r\nAV,120,1,2\r\nAV,120,1,2\r\nAV,120,1,2\r\nAV,120,1,2\r\nAV,120,1,2\r\nAV,120,1,2\r\nAV,120,1,2\r\nAV,120,1,2\r\nAV,120,1,2\r\nAV,120,1,2\r\nAV,120,1,2\r\nAV,120,1,2\r\nAV,120,1,2\r\nAV,120,1,2\r\nAV,120,1,2\r\nAV,120,1,2\r\nAV,120,1,2\r\nAV,120,1,2\r\nAV,120,1,2\r\nAV,120,1,2\r\nAV,120,1,2\r\nAV,120,1,2\r\nAV,120,1,2\r\nAV,120,1,2\r\nAV,120,1,2\r\nAV,120,1,2\r\nAV,120,1,2\r\nAV,120,1,2\r\nAV,120,1,2\r\nAV,120,1,2\r\nAV,120,1,2\r\nAV,120,1,2\r\nAV,120,1,2\r\nAV,120,1,2\r\nAV,120,1,2\r\nAV,120,1,2\r\nAV,120,1,2\r\nAV,120,1,2\r\nAV,120,1,2\r\nAV,120,1,2\r\nAV,120,1,2\r\nAV,120,1,2\r\nAV,120,1,2\r\nAV,120,1,2\r\nAV,120,1,2\r\nAV,120,1,2\r\nAV,120,1,2\r\nAV,120,1,2\r\nAV,120,1,2\r\nAV,120,1,2\r\nAV,120,1,2\r\nAV,120,1,2\r\nAV,120,1,2\r\nAV,120,1,2\r\nAV,120,1,2\r\nAV,120,1,2\r\nAV,120,1,2\r\nAV,120,1,2\r\nAV,120,1,2\r\nAV,120,1,2\r\nAV,120,1,2\r\nAV,120,1,2\r\nAV,120,1,2\r\nAV,120,1,2\r\nAV,120,1,2\r\nAV,120,1,2\r\nAV,120,1,2\r\nAV,120,1,2\r\nAV,120,1,2\r\nAV,120,1,2\r\nAV,120,1,2\r\nAV,120,1,2\r\nAV,120,1,2\r\nAV,120,1,2\r\nAV,120,1,2\r\nAV,120,1,2\r\nAV,120,1,2\r\nAV,120,1,2\r\nAV,120,1,2\r\nAV,120,1,2\r\nAV,120,1,2\r\nAV,120,1,2\r\nAV,120,1,2\r\nAV,120,1,2\r\nAV,120,1,2\r\nAV,120,1,2\r\nAV,120,1,2\r\nAV,120,1,2\r\nAV,120,1,2\r\nAV,120,1,2\r\nAV,120,1,2\r\nAV,120,1,2\r\nAV,120,1,2\r\nAV,120,1,2\r\nAV,120,1,2\r\nAV,120,1,2\r\nAV,120,1,2\r\nAV,120,1,2\r\nAV,120,1,2\r\nAV,120,1,2\r\nAV,120,1,2\r\nAV,120,1,2\r\nAV,120,1,2\r\nAV,120,1,2\r\nAV,120,1,2\r\nAV,120,1,2\r\nAV,120,1,2\r\nAV,120,1,2\r\nAV,120,1,2\r\nAV,120,1,2\r\nAV,120,1,2\r\nAV,120,1,2\r\nAV,120,1,2\r\nAV,120,1,2\r\nAV,120,1,2\r\nAV,120,1,2\r\nAV,120,1,2\r\nAI,400,3,0\r\nAI,400,4,0\r\nAI,400,5,0\r\nAI,401,3,8\r\nAI,401,4,-6\r\nAI,401,5,0\r\nAI,401,3,-8\r\nAI,401,4,-6\r\nAI,401,5,0\r\nAI,401,3,8\r\nAI,401,4,-6\r\nAI,401,5,0\r\nAI,401,3,-8\r\nAI,401,4,-6\r\nAI,401,5,0\r\nAI,401,3,8\r\nAI,401,4,-6\r\nAI,401,5,0\r\nAI,401,3,-8\r\nAI,401,4,-6\r\nAI,401,5,0\r\nAI,401,3,8\r\nAI,401,4,-6\r\nAI,401,5,0\r\nAI,401,3,-8\r\nAI,401,4,-6\r\nAI,401,5,0\r\nAI,401,3,8\r\nAI,401,4,-6\r\nAI,401,5,0\r\nAI,401,3,-8\r\nAI,401,4,-6\r\nAI,401,5,0\r\nAI,401,3,8\r\nAI,401,4,-6\r\nAI,401,5,0\r\nAI,401,3,-8\r\nAI,401,4,-6\r\nAI,401,5,0\r\nAI,401,3,8\r\nAI,401,4,-6\r\nAI,401,5,0\r\nAI,401,3,-8\r\nAI,401,4,-6\r\nAI,401,5,0\r\nAI,401,3,8\r\nAI,401,4,-6\r\nAI,401,5,0\r\nAI,401,3,-8\r\nAI,401,4,-6\r\nAI,401,5,0\r\nAI,401,3,8\r\nAI,401,4,-6\r\nAI,401,5,0\r\nAI,401,3,-8\r\nAI,401,4,-6\r\nAI,401,5,0\r\nAI,401,3,8\r\nAI,401,4,-6\r\nAI,401,5,0\r\nAI,401,3,-8\r\nAI,401,4,-6\r\nAI,401,5,0\r\nAI,401,3,8\r\nAI,401,4,-6\r\nAI,401,5,0\r\nAI,401,3,-8\r\nAI,401,4,-6\r\nAI,401,5,0\r\nAI,401,3,8\r\nAI,401,4,-6\r\nAI,401,5,0\r\nAI,401,3,-8\r\nAI,401,4,-6\r\nAI,401,5,0\r\nAI,401,3,8\r\nAI,401,4,-6\r\nAI,401,5,0\r\nAI,401,3,-8\r\nAI,401,4,-6\r\nAI,401,5,0\r\nAI,401,3,8\r\nAI,401,4,-6\r\nAI,401,5,0\r\nAI,401,3,-8\r\nAI,401,4,-6\r\nAI,401,5,0\r\nAI,401,3,8\r\nAI,401,4,-6\r\nAI,401,5,0\r\nAI,401,3,-8\r\nAI,401,4,-6\r\nAI,401,5,0\r\nAI,401,3,8\r\nAI,401,4,-6\r\nAI,401,5,0\r\nAI,401,3,-8\r\nAI,401,4,-6\r\nAI,401,5,0\r\nAI,401,3,8\r\nAI,401,4,-6\r\nAI,401,5,0\r\nAI,401,3,-8\r\nAI,401,4,-6\r\nAI,401,5,0\r\nAI,401,3,8\r\nAI,401,4,-6\r\nAI,401,5,0\r\nAI,401,3,-8\r\nAI,401,4,-6\r\nAI,401,5,0\r\nAI,401,3,8\r\nAI,401,4,-6\r\nAI,401,5,0\r\nAI,401,3,-8\r\nAI,401,4,-6\r\nAI,401,5,0\r\nAI,401,3,8\r\nAI,401,4,-6\r\nAI,401,5,0\r\nAI,401,3,-8\r\nAI,401,4,-6\r\nAI,401,5,0\r\nAI,401,3,8\r\nAI,401,4,-6\r\nAI,401,5,0\r\nAI,401,3,-8\r\nAI,401,4,-6\r\nAI,401,5,0\r\nAI,401,3,8\r\nAI,401,4,-6\r\nAI,401,5,0\r\nAI,401,3,-8\r\nAI,401,4,-6\r\nAI,401,5,0\r\nAI,401,3,8\r\nAI,401,4,-6\r\nAI,401,5,0\r\nAI,401,3,-8\r\nAI,401,4,-6\r\nAI,401,5,0\r\nAI,401,3,8\r\nAI,401,4,-6\r\nAI,401,5,0\r\nAI,401,3,-8\r\nAI,401,4,-6\r\nAI,401,5,0\r\nAI,401,3,8\r\nAI,401,4,-6\r\nAI,401,5,0\r\nAI,401,3,-8\r\nAI,401,4,-6\r\nAI,401,5,0\r\nAI,401,3,8\r\nAI,401,4,-6\r\nAI,401,5,0\r\nAI,401,3,-8\r\nAI,401,4,-6\r\nAI,401,5,0\r\nAI,401,3,8\r\nAI,401,4,-6\r\nAI,401,5,0\r\nAI,401,3,-8\r\nAI,401,4,-6\r\nAI,401,5,0\r\nAI,401,3,8\r\nAI,401,4,-6\r\nAI,401,5,0\r\nAI,401,3,-8\r\nAI,401,4,-6\r\nAI,401,5,0\r\nAI,401,3,8\r\nAI,401,4,-6\r\nAI,401,5,0\r\nAI,401,3,-8\r\nAI,401,4,-6\r\nAI,401,5,0\r\nAI,401,3,8\r\nAI,401,4,-6\r\nAI,401,5,0\r\nAI,401,3,-8\r\nAI,401,4,-6\r\nAI,401,5,0\r\nAI,401,3,8\r\nAI,401,4,-6\r\nAI,401,5,0\r\nAI,401,3,-8\r\nAI,401,4,-6\r\nAI,401,5,0\r\nAI,401,3,8\r\nAI,401,4,-6\r\nAI,401,5,0\r\nAI,401,3,-8\r\nAI,401,4,-6\r\nAI,401,5,0\r\nAI,401,3,8\r\nAI,401,4,-6\r\nAI,401,5,0\r\nAI,401,3,-8\r\nAI,401,4,-6\r\nAI,401,5,0\r\nAI,401,3,8\r\nAI,401,4,-6\r\nAI,401,5,0\r\nAI,401,3,-8\r\nAI,401,4,-6\r\nAI,401,5,0\r\nAI,401,3,8\r\nAI,401,4,-6\r\nAI,401,5,0\r\nAI,401,3,-8\r\nAI,401,4,-6\r\nAI,401,5,0\r\nAI,401,3,8\r\nAI,401,4,-6\r\nAI,401,5,0\r\nAI,401,3,-8\r\nAI,401,4,-6\r\nAI,401,5,0\r\nAI,401,3,8\r\nAI,401,4,-6\r\nAI,401,5,0\r\nAI,401,3,-8\r\nAI,401,4,-6\r\nAI,401,5,0\r\nAI,401,3,8\r\nAI,401,4,-6\r\nAI,401,5,0\r\nAI,401,3,-8\r\nAI,401,4,-6\r\nAI,401,5,0\r\nAI,401,3,8\r\nAI,401,4,-6\r\nAI,401,5,0\r\nAI,401,3,-8\r\nAI,401,4,-6\r\nAI,401,5,0\r\nAI,401,3,8\r\nAI,401,4,-6\r\nAI,401,5,0\r\nAI,401,3,-8\r\nAI,401,4,-6\r\nAI,401,5,0\r\nAI,401,3,8\r\nAI,401,4,-6\r\nAI,401,5,0\r\nAI,401,3,-8\r\nAI,401,4,-6\r\nAI,401,5,0\r\nAI,401,3,8\r\nAI,401,4,-6\r\nAI,401,5,0\r\nAI,401,3,-8\r\nAI,401,4,-6\r\nAI,401,5,0\r\nAI,401,3,8\r\nAI,401,4,-6\r\nAI,401,5,0\r\nAI,401,3,-8\r\nAI,401,4,-6\r\nAI,401,5,0\r\nAI,401,3,8\r\nAI,401,4,-6\r\nAI,401,5,0\r\nAI,401,3,-8\r\nAI,401,4,-6\r\nAI,401,5,0\r\nAI,401,3,8\r\nAI,401,4,-6\r\nAI,401,5,0\r\nAI,401,3,-8\r\nAI,401,4,-6\r\nAI,401,5,0\r\nAI,401,3,8\r\nAI,401,4,-6\r\nAI,401,5,0\r\nAI,401,3,-8\r\nAI,401,4,-6\r\nAI,401,5,0\r\nAI,401,3,8\r\nAI,401,4,-6\r\nAI,401,5,0\r\nAI,401,3,-8\r\nAI,401,4,-6\r\nAI,401,5,0\r\nAI,401,3,8\r\nAI,401,4,-6\r\nAI,401,5,0\r\nAI,401,3,-8\r\nAI,401,4,-6\r\nAI,401,5,0\r\nAI,401,3,8\r\nAI,401,4,-6\r\nAI,401,5,0\r\nAI,401,3,-8\r\nAI,401,4,-6\r\nAI,401,5,0\r\nAI,401,3,8\r\nAI,401,4,-6\r\nAI,401,5,0\r\nAI,401,3,-8\r\nAI,401,4,-6\r\nAI,401,5,0\r\nAI,401,3,8\r\nAI,401,4,-6\r\nAI,401,5,0\r\nAI,401,3,-8\r\nAI,401,4,-6\r\nAI,401,5,0\r\nAI,401,3,8\r\nAI,401,4,-6\r\nAI,401,5,0\r\nAI,401,3,-8\r\nAI,401,4,-6\r\nAI,401,5,0\r\nAI,401,3,8\r\nAI,401,4,-6\r\nAI,401,5,0\r\nAI,401,3,-8\r\nAI,401,4,-6\r\nAI,401,5,0\r\nAI,401,3,8\r\nAI,401,4,-6\r\nAI,401,5,0\r\nAI,401,3,-8\r\nAI,401,4,-6\r\nAI,401,5,0\r\nAI,401,3,8\r\nAI,401,4,-6\r\nAI,401,5,0\r\nAI,401,3,-8\r\nAI,401,4,-6\r\nAI,401,5,0\r\nAI,401,3,8\r\nAI,401,4,-6\r\nAI,401,5,0\r\nAI,401,3,-8\r\nAI,401,4,-6\r\nAI,401,5,0\r\nAI,401,3,8\r\nAI,401,4,-6\r\nAI,401,5,0\r\nAI,401,3,-8\r\nAI,401,4,-6\r\nAI,401,5,0\r\nAI,401,3,8\r\nAI,401,4,-6\r\nAI,401,5,0\r\nAI,401,3,-8\r\nAI,401,4,-6\r\nAI,401,5,0\r\nAI,401,3,8\r\nAI,401,4,-6\r\nAI,401,5,0\r\nAI,401,3,-8\r\nAI,401,4,-6\r\nAI,401,5,0\r\nAI,401,3,8\r\nAI,401,4,-6\r\nAI,401,5,0\r\nAI,401,3,-8\r\nAI,401,4,-6\r\nAI,401,5,0\r\nAI,401,3,8\r\nAI,401,4,-6\r\nAI,401,5,0\r\nAI,401,3,-8\r\nAI,401,4,-6\r\nAI,401,5,0\r\nAI,401,3,8\r\nAI,401,4,-6\r\nAI,401,5,0\r\nAI,401,3,-8\r\nAI,401,4,-6\r\nAI,401,5,0\r\nAI,401,3,8\r\nAI,401,4,-6\r\nAI,401,5,0\r\nAI,401,3,-8\r\nAI,401,4,-6\r\nAI,401,5,0\r\nAI,401,3,8\r\nAI,401,4,-6\r\nAI,401,5,0\r\nAI,401,3,-8\r\nAI,401,4,-6\r\nAI,401,5,0\r\nAI,401,3,8\r\nAI,401,4,-6\r\nAI,401,5,0\r\nAI,401,3,-8\r\nAI,401,4,-6\r\nAI,401,5,0\r\nAI,401,3,8\r\nAI,401,4,-6\r\nAI,401,5,0\r\nAI,401,3,-8\r\nAI,401,4,-6\r\nAI,401,5,0\r\nAI,401,3,8\r\nAI,401,4,-6\r\nAI,401,5,0\r\nAI,401,3,-8\r\nAI,401,4,-6\r\nAI,401,5,0\r\nAI,401,3,8\r\nAI,401,4,-6\r\nAI,401,5,0\r\nAI,401,3,-8\r\nAI,401,4,-6\r\nAI,401,5,0\r\nAI,401,3,8\r\nAI,401,4,-6\r\nAI,401,5,0\r\nAI,401,3,-8\r\nAI,401,4,-6\r\nAI,401,5,0\r\nAI,401,3,8\r\nAI,401,4,-6\r\nAI,401,5,0\r\nAI,401,3,-8\r\nAI,401,4,-6\r\nAI,401,5,0\r\nAI,401,3,8\r\nAI,401,4,-6\r\nAI,401,5,0\r\nAI,401,3,-8\r\nAI,401,4,-6\r\nAI,401,5,0\r\nAI,401,3,8\r\nAI,401,4,-6\r\nAI,401,5,0\r\nAI,401,3,-8\r\nAI,401,4,-6\r\nAI,401,5,0\r\nAI,401,3,8\r\nAI,401,4,-6\r\nAI,401,5,0\r\nAI,401,3,-8\r\nAI,401,4,-6\r\nAI,401,5,0\r\nAI,401,3,8\r\nAI,401,4,-6\r\nAI,401,5,0\r\nAI,401,3,-8\r\nAI,401,4,-6\r\nAI,401,5,0\r\nAI,401,3,8\r\nAI,401,4,-6\r\nAI,401,5,0\r\nAI,401,3,-8\r\nAI,401,4,-6\r\nAI,401,5,0\r\nAI,401,3,8\r\nAI,401,4,-6\r\nAI,401,5,0\r\nAI,401,3,-8\r\nAI,401,4,-6\r\nAI,401,5,0\r\nAI,401,3,8\r\nAI,401,4,-6\r\nAI,401,5,0\r\nAI,401,3,-8\r\nAI,401,4,-6\r\nAI,401,5,0\r\nAI,401,3,8\r\nAI,401,4,-6\r\nAI,401,5,0\r\nAI,401,3,-8\r\nAI,401,4,-6\r\nAI,401,5,0\r\nAI,401,3,8\r\nAI,401,4,-6\r\nAI,401,5,0\r\nAI,401,3,-8\r\nAI,401,4,-6\r\nAI,401,5,0\r\nAI,401,3,8\r\nAI,401,4,-6\r\nAI,401,5,0\r\nAI,401,3,-8\r\nAI,401,4,-6\r\nAI,401,5,0\r\nAI,401,3,8\r\nAI,401,4,-6\r\nAI,401,5,0\r\nAI,401,3,-8\r\nAI,401,4,-6\r\nAI,401,5,0\r\nAI,401,3,8\r\nAI,401,4,-6\r\nAI,401,5,0\r\nAI,401,3,-8\r\nAI,401,4,-6\r\nAI,401,5,0\r\nAI,401,3,8\r\nAI,401,4,-6\r\nAI,401,5,0\r\nAI,401,3,-8\r\nAI,401,4,-6\r\nAI,401,5,0\r\nAI,401,3,8\r\nAI,401,4,-6\r\nAI,401,5,0\r\nAI,401,3,-8\r\nAI,401,4,-6\r\nAI,401,5,0\r\nAI,401,3,8\r\nAI,401,4,-6\r\nAI,401,5,0\r\nAI,401,3,-8\r\nAI,401,4,-6\r\nAI,401,5,0\r\nAI,401,3,8\r\nAI,401,4,-6\r\nAI,401,5,0\r\nAI,401,3,-8\r\nAI,401,4,-6\r\nAI,401,5,0\r\nAI,401,3,8\r\nAI,401,4,-6\r\nAI,401,5,0\r\nAI,401,3,-8\r\nAI,401,4,-6\r\nAI,401,5,0\r\nAI,401,3,8\r\nAI,401,4,-6\r\nAI,401,5,0\r\nAI,401,3,-8\r\nAI,401,4,-6\r\nAI,401,5,0\r\nAI,401,3,8\r\nAI,401,4,-6\r\nAI,401,5,0\r\nAI,401,3,-8\r\nAI,401,4,-6\r\nAI,401,5,0\r\nAI,401,3,8\r\nAI,401,4,-6\r\nAI,401,5,0\r\nAI,401,3,-8\r\nAI,401,4,-6\r\nAI,401,5,0\r\nAI,401,3,8\r\nAI,401,4,-6\r\nAI,401,5,0\r\nAI,401,3,-8\r\nAI,401,4,-6\r\nAI,401,5,0\r\nAI,401,3,8\r\nAI,401,4,-6\r\nAI,401,5,0\r\nAI,401,3,-8\r\nAI,401,4,-6\r\nAI,401,5,0\r\nAI,401,3,8\r\nAI,401,4,-6\r\nAI,401,5,0\r\nAI,401,3,-8\r\nAI,401,4,-6\r\nAI,401,5,0\r\nAI,401,3,8\r\nAI,401,4,-6\r\nAI,401,5,0\r\nAI,401,3,-8\r\nAI,401,4,-6\r\nAI,401,5,0\r\nAI,401,3,8\r\nAI,401,4,-6\r\nAI,401,5,0\r\nAI,401,3,-8\r\nAI,401,4,-6\r\nAI,401,5,0\r\nAI,401,3,8\r\nAI,401,4,-6\r\nAI,401,5,0\r\nAI,401,3,-8\r\nAI,401,4,-6\r\nAI,401,5,0\r\nAI,401,3,8\r\nAI,401,4,-6\r\nAI,401,5,0\r\nAI,401,3,-8\r\nAI,401,4,-6\r\nAI,401,5,0\r\nAI,401,3,8\r\nAI,401,4,-6\r\nAI,401,5,0\r\nAI,401,3,-8\r\nAI,401,4,-6\r\nAI,401,5,0\r\nAI,401,3,8\r\nAI,401,4,-6\r\nAI,401,5,0\r\nAI,401,3,-8\r\nAI,401,4,-6\r\nAI,401,5,0\r\nAI,401,3,8\r\nAI,401,4,-6\r\nAI,401,5,0\r\nAI,401,3,-8\r\nAI,401,4,-6\r\nAI,401,5,0\r\nAI,401,3,8\r\nAI,401,4,-6\r\nAI,401,5,0\r\nAI,401,3,-8\r\nAI,401,4,-6\r\nAI,401,5,0\r\nAI,401,3,8\r\nAI,401,4,-6\r\nAI,401,5,0\r\nAI,401,3,-8\r\nAI,401,4,-6\r\nAI,401,5,0\r\nAI,401,3,8\r\nAI,401,4,-6\r\nAI,401,5,0\r\nAI,401,3,-8\r\nAI,401,4,-6\r\nAI,401,5,0\r\nAI,401,3,8\r\nAI,401,4,-6\r\nAI,401,5,0\r\nAI,401,3,-8\r\nAI,401,4,-6\r\nAI,401,5,0\r\nAI,401,3,8\r\nAI,401,4,-6\r\nAI,401,5,0\r\nAI,401,3,-8\r\nAI,401,4,-6\r\nAI,401,5,0\r\nAI,401,3,8\r\nAI,401,4,-6\r\nAI,401,5,0\r\nAI,401,3,-8\r\nAI,401,4,-6\r\nAI,401,5,0\r\nAI,401,3,8\r\nAI,401,4,-6\r\nAI,401,5,0\r\nAI,401,3,-8\r\nAI,401,4,-6\r\nAI,401,5,0\r\nAI,401,3,8\r\nAI,401,4,-6\r\nAI,401,5,0\r\nAI,401,3,-8\r\nAI,401,4,-6\r\nAI,401,5,0\r\nAI,401,3,8\r\nAI,401,4,-6\r\nAI,401,5,0\r\nAI,401,3,-8\r\nAI,401,4,-6\r\nAI,401,5,0\r\nAI,401,3,8\r\nAI,401,4,-6\r\nAI,401,5,0\r\nAI,401,3,-8\r\nAI,401,4,-6\r\nAI,401,5,0\r\nAI,401,3,8\r\nAI,401,4,-6\r\nAI,401,5,0\r\nAI,401,3,-8\r\nAI,401,4,-6\r\nAI,401,5,0\r\nAI,401,3,8\r\nAI,401,4,-6\r\nAI,401,5,0\r\nAI,401,3,-8\r\nAI,401,4,-6\r\nAI,401,5,0\r\nAI,401,3,8\r\nAI,401,4,-6\r\nAI,401,5,0\r\nAI,401,3,-8\r\nAI,401,4,-6\r\nAI,401,5,0\r\nAI,401,3,8\r\nAI,401,4,-6\r\nAI,401,5,0\r\nAI,401,3,-8\r\nAI,401,4,-6\r\nAI,401,5,0\r\nAI,401,3,8\r\nAI,401,4,-6\r\nAI,401,5,0\r\nAI,401,3,-8\r\nAI,401,4,-6\r\nAI,401,5,0\r\nAI,401,3,8\r\nAI,401,4,-6\r\nAI,401,5,0\r\nAI,401,3,-8\r\nAI,401,4,-6\r\nAI,401,5,0\r\nAI,401,3,8\r\nAI,401,4,-6\r\nAI,401,5,0\r\nAI,401,3,-8\r\nAI,401,4,-6\r\nAI,401,5,0\r\nAI,401,3,8\r\nAI,401,4,-6\r\nAI,401,5,0\r\nAI,401,3,-8\r\nAI,401,4,-6\r\nAI,401,5,0\r\nAI,401,3,8\r\nAI,401,4,-6\r\nAI,401,5,0\r\nAI,401,3,-8\r\nAI,401,4,-6\r\nAI,401,5,0\r\nAI,401,3,8\r\nAI,401,4,-6\r\nAI,401,5,0\r\nAI,401,3,-8\r\nAI,401,4,-6\r\nAI,401,5,0\r\nAI,401,3,8\r\nAI,401,4,-6\r\nAI,401,5,0\r\nAI,401,3,-8\r\nAI,401,4,-6\r\nAI,401,5,0\r\nAI,401,3,8\r\nAI,401,4,-6\r\nAI,401,5,0\r\nAI,401,3,-8\r\nAI,401,4,-6\r\nAI,401,5,0\r\nAI,401,3,8\r\nAI,401,4,-6\r\nAI,401,5,0\r\nAI,401,3,-8\r\nAI,401,4,-6\r\nAI,401,5,0\r\nAI,401,3,8\r\nAI,401,4,-6\r\nAI,401,5,0\r\nAI,401,3,-8\r\nAI,401,4,-6\r\nAI,401,5,0\r\nAI,401,3,8\r\nAI,401,4,-6\r\nAI,401,5,0\r\nAI,401,3,-8\r\nAI,401,4,-6\r\nAI,401,5,0\r\nAI,401,3,8\r\nAI,401,4,-6\r\nAI,401,5,0\r\nAI,401,3,-8\r\nAI,401,4,-6\r\nAI,401,5,0\r\nAI,401,3,8\r\nAI,401,4,-6\r\nAI,401,5,0\r\nAI,401,3,-8\r\nAI,401,4,-6\r\nAI,401,5,0\r\nAI,401,3,8\r\nAI,401,4,-6\r\nAI,401,5,0\r\nAI,401,3,-8\r\nAI,401,4,-6\r\nAI,401,5,0\r\nAI,401,3,8\r\nAI,401,4,-6\r\nAI,401,5,0\r\nAI,401,3,-8\r\nAI,401,4,-6\r\nAI,401,5,0\r\nAI,401,3,8\r\nAI,401,4,-6\r\nAI,401,5,0\r\nAI,401,3,-8\r\nAI,401,4,-6\r\nAI,401,5,0\r\nAI,401,3,8\r\nAI,401,4,-6\r\nAI,401,5,0\r\nAI,401,3,-8\r\nAI,401,4,-6\r\nAI,401,5,0\r\nAI,401,3,8\r\nAI,401,4,-6\r\nAI,401,5,0\r\nAI,401,3,-8\r\nAI,401,4,-6\r\nAI,401,5,0\r\nAI,401,3,8\r\nAI,401,4,-6\r\nAI,401,5,0\r\nAI,401,3,-8\r\nAI,401,4,-6\r\nAI,401,5,0\r\nAI,401,3,8\r\nAI,401,4,-6\r\nAI,401,5,0\r\nAI,401,3,-8\r\nAI,401,4,-6\r\nAI,401,5,0\r\nAI,401,3,8\r\nAI,401,4,-6\r\nAI,401,5,0\r\nAI,401,3,-8\r\nAI,401,4,-6\r\nAI,401,5,0\r\nAI,401,3,8\r\nAI,401,4,-6\r\nAI,401,5,0\r\nAI,401,3,-8\r\nAI,401,4,-6\r\nAI,401,5,0\r\nAI,401,3,8\r\nAI,401,4,-6\r\nAI,401,5,0\r\nAI,401,3,-8\r\nAI,401,4,-6\r\nAI,401,5,0\r\nAI,401,3,8\r\nAI,401,4,-6\r\nAI,401,5,0\r\nAI,401,3,-8\r\nAI,401,4,-6\r\nAI,401,5,0\r\nAI,401,3,8\r\nAI,401,4,-6\r\nAI,401,5,0\r\nAI,401,3,-8\r\nAI,401,4,-6\r\nAI,401,5,0\r\nAI,401,3,8\r\nAI,401,4,-6\r\nAI,401,5,0\r\nAI,401,3,-8\r\nAI,401,4,-6\r\nAI,401,5,0\r\nAI,401,3,8\r\nAI,401,4,-6\r\nAI,401,5,0\r\nAI,401,3,-8\r\nAI,401,4,-6\r\nAI,401,5,0\r\nAI,401,3,8\r\nAI,401,4,-6\r\nAI,401,5,0\r\nAI,401,3,-8\r\nAI,401,4,-6\r\nAI,401,5,0\r\nAI,401,3,8\r\nAI,401,4,-6\r\nAI,401,5,0\r\nAI,401,3,-8\r\nAI,401,4,-6\r\nAI,401,5,0\r\nAI,401,3,8\r\nAI,401,4,-6\r\nAI,401,5,0\r\nAI,401,3,-8\r\nAI,401,4,-6\r\nAI,401,5,0\r\nAI,401,3,8\r\nAI,401,4,-6\r\nAI,401,5,0\r\nAI,401,3,-8\r\nAI,401,4,-6\r\nAI,401,5,0\r\nAI,401,3,8\r\nAI,401,4,-6\r\nAI,401,5,0\r\nAI,401,3,-8\r\nAI,401,4,-6\r\nAI,401,5,0\r\nAI,401,3,8\r\nAI,401,4,-6\r\nAI,401,5,0\r\nAI,401,3,-8\r\nAI,401,4,-6\r\nAI,401,5,0\r\nAI,401,3,8\r\nAI,401,4,-6\r\nAI,401,5,0\r\nAI,401,3,-8\r\nAI,401,4,-6\r\nAI,401,5,0\r\nAI,401,3,8\r\nAI,401,4,-6\r\nAI,401,5,0\r\nAI,401,3,-8\r\nAI,401,4,-6\r\nAI,401,5,0\r\nAI,401,3,8\r\nAI,401,4,-6\r\nAI,401,5,0\r\nAI,401,3,-8\r\nAI,401,4,-6\r\nAI,401,5,0\r\nAI,401,3,8\r\nAI,401,4,-6\r\nAI,401,5,0\r\nAI,401,3,-8\r\nAI,401,4,-6\r\nAI,401,5,0\r\nAI,401,3,8\r\nAI,401,4,-6\r\nAI,401,5,0\r\nAI,401,3,-8\r\nAI,401,4,-6\r\nAI,401,5,0\r\nAI,401,3,8\r\nAI,401,4,-6\r\nAI,401,5,0\r\nAI,401,3,-8\r\nAI,401,4,-6\r\nAI,401,5,0\r\nAI,401,3,8\r\nAI,401,4,-6\r\nAI,401,5,0\r\nAI,401,3,-8\r\nAI,401,4,-6\r\nAI,401,5,0\r\nAI,401,3,8\r\nAI,401,4,-6\r\nAI,401,5,0\r\nAI,401,3,-8\r\nAI,401,4,-6\r\nAI,401,5,0\r\nAI,401,3,8\r\nAI,401,4,-6\r\nAI,401,5,0\r\nAI,401,3,-8\r\nAI,401,4,-6\r\nAI,401,5,0\r\nAI,401,3,8\r\nAI,401,4,-6\r\nAI,401,5,0\r\nAI,401,3,-8\r\nAI,401,4,-6\r\nAI,401,5,0\r\nAI,401,3,8\r\nAI,401,4,-6\r\nAI,401,5,0\r\nAI,401,3,-8\r\nAI,401,4,-6\r\nAI,401,5,0\r\nAI,401,3,8\r\nAI,401,4,-6\r\nAI,401,5,0\r\nAI,401,3,-8\r\nAI,401,4,-6\r\nAI,401,5,0\r\nAI,401,3,8\r\nAI,401,4,-6\r\nAI,401,5,0\r\nAI,401,3,-8\r\nAI,401,4,-6\r\nAI,401,5,0\r\nAI,401,3,8\r\nAI,401,4,-6\r\nAI,401,5,0\r\nAI,401,3,-8\r\nAI,401,4,-6\r\nAI,401,5,0\r\nAI,401,3,8\r\nAI,401,4,-6\r\nAI,401,5,0\r\nAI,401,3,-8\r\nAI,401,4,-6\r\nAI,401,5,0\r\nAI,401,3,8\r\nAI,401,4,-6\r\nAI,401,5,0\r\nAI,401,3,-8\r\nAI,401,4,-6\r\nAI,401,5,0\r\nAI,401,3,8\r\nAI,401,4,-6\r\nAI,401,5,0\r\nAI,401,3,-8\r\nAI,401,4,-6\r\nAI,401,5,0\r\nAI,401,3,8\r\nAI,401,4,-6\r\nAI,401,5,0\r\nAI,401,3,-8\r\nAI,401,4,-6\r\nAI,401,5,0\r\nAI,401,3,8\r\nAI,401,4,-6\r\nAI,401,5,0\r\nAI,401,3,-8\r\nAI,401,4,-6\r\nAI,401,5,0\r\nAI,401,3,8\r\nAI,401,4,-6\r\nAI,401,5,0\r\nAI,401,3,-8\r\nAI,401,4,-6\r\nAI,401,5,0\r\nAI,401,3,8\r\nAI,401,4,-6\r\nAI,401,5,0\r\nAI,401,3,-8\r\nAI,401,4,-6\r\nAI,401,5,0\r\nAI,401,3,8\r\nAI,401,4,-6\r\nAI,401,5,0\r\nAI,401,3,-8\r\nAI,401,4,-6\r\nAI,401,5,0\r\nAI,401,3,8\r\nAI,401,4,-6\r\nAI,401,5,0\r\nAI,401,3,-8\r\nAI,401,4,-6\r\nAI,401,5,0\r\nAI,401,3,8\r\nAI,401,4,-6\r\nAI,401,5,0\r\nAI,401,3,-8\r\nAI,401,4,-6\r\nAI,401,5,0\r\nAI,401,3,8\r\nAI,401,4,-6\r\nAI,401,5,0\r\nAI,401,3,-8\r\nAI,401,4,-6\r\nAI,401,5,0\r\nAI,401,3,8\r\nAI,401,4,-6\r\nAI,401,5,0\r\nAI,401,3,-8\r\nAI,401,4,-6\r\nAI,401,5,0\r\nAI,401,3,8\r\nAI,401,4,-6\r\nAI,401,5,0\r\nAI,401,3,-8\r\nAI,401,4,-6\r\nAI,401,5,0\r\nAI,401,3,8\r\nAI,401,4,-6\r\nAI,401,5,0\r\nAI,401,3,-8\r\nAI,401,4,-6\r\nAI,401,5,0\r\nAI,401,3,8\r\nAI,401,4,-6\r\nAI,401,5,0\r\nAI,401,3,-8\r\nAI,401,4,-6\r\nAI,401,5,0\r\nAI,401,3,8\r\nAI,401,4,-6\r\nAI,401,5,0\r\nAI,401,3,-8\r\nAI,401,4,-6\r\nAI,401,5,0\r\nAI,401,3,8\r\nAI,401,4,-6\r\nAI,401,5,0\r\nAI,401,3,-8\r\nAI,401,4,-6\r\nAI,401,5,0\r\nAI,401,3,8\r\nAI,401,4,-6\r\nAI,401,5,0\r\nAI,401,3,-8\r\nAI,401,4,-6\r\nAI,401,5,0\r\nAI,401,3,8\r\nAI,401,4,-6\r\nAI,401,5,0\r\nAI,401,3,-8\r\nAI,401,4,-6\r\nAI,401,5,0\r\nAI,401,3,8\r\nAI,401,4,-6\r\nAI,401,5,0\r\nAI,401,3,-8\r\nAI,401,4,-6\r\nAI,401,5,0\r\nAI,401,3,8\r\nAI,401,4,-6\r\nAI,401,5,0\r\nAI,401,3,-8\r\nAI,401,4,-6\r\nAI,401,5,0\r\nAI,401,3,8\r\nAI,401,4,-6\r\nAI,401,5,0\r\nAI,401,3,-8\r\nAI,401,4,-6\r\nAI,401,5,0\r\nAI,401,3,8\r\nAI,401,4,-6\r\nAI,401,5,0\r\nAI,401,3,-8\r\nAI,401,4,-6\r\nAI,401,5,0\r\nAI,401,3,8\r\nAI,401,4,-6\r\nAI,401,5,0\r\nAI,401,3,-8\r\nAI,401,4,-6\r\nAI,401,5,0\r\nAI,401,3,8\r\nAI,401,4,-6\r\nAI,401,5,0\r\nAI,401,3,-8\r\nAI,401,4,-6\r\nAI,401,5,0\r\nAI,401,3,8\r\nAI,401,4,-6\r\nAI,401,5,0\r\nAI,401,3,-8\r\nAI,401,4,-6\r\nAI,401,5,0\r\nAI,401,3,8\r\nAI,401,4,-6\r\nAI,401,5,0\r\nAI,401,3,-8\r\nAI,401,4,-6\r\nAI,401,5,0\r\nAI,401,3,8\r\nAI,401,4,-6\r\nAI,401,5,0\r\nAI,401,3,-8\r\nAI,401,4,-6\r\nAI,401,5,0\r\nAI,401,3,8\r\nAI,401,4,-6\r\nAI,401,5,0\r\nAI,401,3,-8\r\nAI,401,4,-6\r\nAI,401,5,0\r\nAI,401,3,8\r\nAI,401,4,-6\r\nAI,401,5,0\r\nAI,401,3,-8\r\nAI,401,4,-6\r\nAI,401,5,0\r\nAI,401,3,8\r\nAI,401,4,-6\r\nAI,401,5,0\r\nAI,401,3,-8\r\nAI,401,4,-6\r\nAI,401,5,0\r\nAI,401,3,8\r\nAI,401,4,-6\r\nAI,401,5,0\r\nAI,401,3,-8\r\nAI,401,4,-6\r\nAI,401,5,0\r\nAI,401,3,8\r\nAI,401,4,-6\r\nAI,401,5,0\r\nAI,401,3,-8\r\nAI,401,4,-6\r\nAI,401,5,0\r\nAI,401,3,8\r\nAI,401,4,-6\r\nAI,401,5,0\r\nAI,401,3,-8\r\nAI,401,4,-6\r\nAI,401,5,0\r\nAI,401,3,8\r\nAI,401,4,-6\r\nAI,401,5,0\r\nAI,401,3,-8\r\nAI,401,4,-6\r\nAI,401,5,0\r\nAI,401,3,8\r\nAI,401,4,-6\r\nAI,401,5,0\r\nAI,401,3,-8\r\nAI,401,4,-6\r\nAI,401,5,0\r\nAI,401,3,8\r\nAI,401,4,-6\r\nAI,401,5,0\r\nAI,401,3,-8\r\nAI,401,4,-6\r\nAI,401,5,0\r\nAI,401,3,8\r\nAI,401,4,-6\r\nAI,401,5,0\r\nAI,401,3,-8\r\nAI,401,4,-6\r\nAI,401,5,0\r\nAI,401,3,8\r\nAI,401,4,-6\r\nAI,401,5,0\r\nAV,520,1,0\r\nAV,521,1,3\r\nAV,521,1,3\r\nAV,521,1,3\r\nAV,521,1,3\r\nAV,521,1,3\r\nAV,521,1,3\r\nAV,521,1,3\r\nAV,521,1,3\r\nAV,521,1,3\r\nAV,521,1,3\r\nAV,521,1,3\r\nAV,521,1,3\r\nAV,521,1,3\r\nAV,521,1,3\r\nAV,521,1,3\r\nAV,521,1,3\r\nAV,521,1,3\r\nAV,521,1,3\r\nAV,521,1,3\r\nAV,521,1,3\r\nAV,521,1,3\r\nAV,521,1,3\r\nAV,521,1,3\r\nAV,521,1,3\r\nAV,521,1,3\r\nAV,521,1,3\r\nAV,521,1,3\r\nAV,521,1,3\r\nAV,521,1,3\r\nAV,521,1,3\r\nAV,521,1,3\r\nAV,521,1,3\r\nAV,521,1,3\r\nAV,521,1,3\r\nAV,521,1,3\r\nAV,521,1,3\r\nAV,521,1,3\r\nAV,521,1,3\r\nAV,521,1,3\r\nAV,521,1,3\r\nAV,521,1,3\r\nAV,521,1,3\r\nAV,521,1,3\r\nAV,521,1,3\r\nAV,521,1,3\r\nAV,521,1,3\r\nAV,521,1,3\r\nAV,521,1,3\r\nAV,521,1,3\r\nAV,521,1,3\r\nAV,521,1,3\r\nAV,521,1,3\r\nAV,521,1,3\r\nAV,521,1,3\r\nAV,521,1,3\r\nAV,521,1,3\r\nAV,521,1,3\r\nAV,521,1,3\r\nAV,521,1,3\r\nAV,521,1,3\r\nAV,521,1,3\r\nAV,521,1,3\r\nAV,521,1,3\r\nAV,521,1,3\r\nAV,521,1,3\r\nAV,521,1,3\r\nAV,521,1,3\r\nAV,521,1,3\r\nAV,521,1,3\r\nAV,521,1,3\r\nAV,521,1,3\r\nAV,521,1,3\r\nAV,521,1,3\r\nAV,521,1,3\r\nAV,521,1,3\r\nAV,521,1,3\r\nAV,521,1,3\r\nAV,521,1,3\r\nAV,521,1,3\r\nAV,521,1,3\r\nAV,521,1,3\r\nAV,521,1,3\r\nAV,521,1,3\r\nAV,521,1,3\r\nAV,521,1,3\r\nAV,521,1,3\r\nAV,521,1,3\r\nAV,521,1,3\r\nAV,521,1,3\r\nAV,521,1,3\r\nAV,521,1,3\r\nAV,521,1,3\r\nAV,521,1,3\r\nAV,521,1,3\r\nAV,521,1,3\r\nAV,521,1,3\r\nAV,521,1,3\r\nAV,521,1,3\r\nAV,521,1,3\r\nAV,521,1,3\r\nAV,521,1,3\r\nAV,521,1,3\r\nAV,521,1,3\r\nAV,521,1,3\r\nAV,521,1,3\r\nAV,521,1,3\r\nAV,521,1,3\r\nAV,521,1,3\r\nAV,521,1,3\r\nAV,521,1,3\r\nAV,521,1,3\r\nAV,521,1,3\r\nAV,521,1,3\r\nAV,521,1,3\r\nAV,521,1,3\r\nAV,521,1,3\r\nAV,521,1,3\r\nAV,521,1,3\r\nAV,521,1,3\r\nAV,521,1,3\r\nAV,521,1,3\r\nAV,521,1,3\r\nAV,521,1,3\r\nAV,521,1,3\r\nAV,521,1,3\r\nAV,521,1,3\r\nAV,521,1,3\r\nAV,521,1,3\r\nAV,521,1,3\r\nAV,521,1,3\r\nAV,521,1,3\r\nAV,521,1,3\r\nAV,521,1,3\r\nAV,521,1,3\r\nAV,521,1,3\r\nAV,521,1,3\r\nAV,521,1,3\r\nAV,521,1,3\r\nAV,521,1,3\r\nAV,521,1,3\r\nAV,521,1,3\r\nAV,521,1,3\r\nAV,521,1,3\r\nAV,521,1,3\r\nAV,521,1,3\r\nAV,521,1,3\r\nAV,521,1,3\r\nAV,521,1,3\r\nAV,521,1,3\r\nAV,521,1,3\r\nAV,521,1,3\r\nAV,521,1,3\r\nAV,521,1,3\r\nAV,521,1,3\r\nAV,521,1,3\r\nAV,521,1,3\r\nAV,521,1,3\r\nAV,521,1,3\r\nAV,521,1,3\r\nAV,521,1,3\r\nAV,521,1,3\r\nAV,521,1,3\r\nAV,521,1,3\r\nAV,521,1,3\r\nAV,521,1,3\r\nAV,521,1,3\r\nAV,521,1,3\r\nAV,521,1,3\r\nAV,521,1,3\r\nAV,521,1,3\r\nAV,521,1,3\r\nAV,521,1,3\r\nAV,521,1,3\r\nAV,521,1,3\r\nAV,521,1,3\r\nAV,521,1,3\r\nAV,521,1,3\r\nAV,521,1,3\r\nAV,521,1,3\r\nAV,521,1,3\r\nAV,521,1,3\r\nAV,521,1,3\r\nAV,521,1,3\r\nAV,521,1,3\r\nAV,521,1,3\r\nAV,521,1,3\r\nAV,521,1,3\r\nAV,521,1,3\r\nAV,521,1,3\r\nAV,521,1,3\r\nAV,521,1,3\r\nAV,521,1,3\r\nAV,521,1,3\r\nAV,521,1,3\r\nAV,521,1,3\r\nAV,521,1,3\r\nAV,521,1,3\r\nAV,521,1,3\r\nAV,521,1,3\r\nAV,521,1,3\r\nAV,521,1,3\r\nAV,521,1,3\r\nAV,521,1,3\r\nAV,521,1,3\r\nAV,521,1,3\r\nAV,521,1,3\r\nAV,521,1,3\r\nAV,521,1,3\r\nAV,521,1,3\r\nAV,521,1,3\r\nAV,521,1,3\r\nAV,521,1,3\r\nAV,521,1,3\r\nAV,521,1,3\r\nAV,521,1,3\r\nAV,521,1,3\r\nAV,521,1,3\r\nAV,521,1,3\r\nAV,521,1,3\r\nAV,521,1,3\r\nAV,521,1,3\r\nAV,521,1,3\r\nAV,521,1,3\r\nAV,521,1,3\r\nAV,521,1,3\r\nAV,521,1,3\r\nAV,521,1,3\r\nAV,521,1,3\r\nAV,521,1,3\r\nAV,521,1,3\r\nAV,521,1,3\r\nAV,521,1,3\r\nAV,521,1,3\r\nAV,521,1,3\r\nAV,521,1,3\r\nAV,521,1,3\r\nAV,521,1,3\r\nAV,521,1,3\r\nAV,521,1,3\r\nAV,521,1,3\r\nAV,521,1,3\r\nAV,521,1,3\r\nAV,521,1,3\r\nAV,521,1,3\r\nAV,521,1,3\r\nAV,521,1,3\r\nAV,521,1,3\r\nAV,521,1,3\r\nAV,521,1,3\r\nAV,521,1,3\r\nAV,521,1,3\r\nAV,521,1,3\r\nAV,521,1,3\r\nAV,521,1,3\r\nAV,521,1,3\r\nAV,521,1,3\r\nAV,521,1,3\r\nAV,521,1,3\r\nAV,521,1,3\r\nAV,521,1,3\r\nAV,521,1,3\r\nAV,521,1,3\r\nAV,521,1,3\r\nAV,521,1,3\r\nAV,521,1,3\r\nAV,521,1,3\r\nAV,521,1,3\r\nAV,521,1,3\r\nAV,521,1,3\r\nAV,521,1,3\r\nAV,521,1,3\r\nAV,521,1,3\r\nAV,521,1,3\r\nAV,521,1,3\r\nAV,521,1,3\r\nAV,521,1,3\r\nAV,521,1,3\r\nAV,521,1,3\r\nAV,521,1,3\r\nAV,521,1,3\r\nAV,521,1,3\r\nAV,521,1,3\r\nAV,521,1,3\r\nAV,521,1,3\r\nAV,521,1,3\r\nAV,521,1,3\r\nAV,521,1,3\r\nAV,521,1,3\r\nAV,521,1,3\r\nAV,521,1,3\r\nAV,521,1,3\r\nAV,521,1,3\r\nAV,521,1,3\r\nAV,521,1,3\r\nAV,521,1,3\r\nAV,521,1,3\r\nAV,521,1,3\r\nAV,521,1,3\r\nAV,521,1,3\r\nAV,521,1,3\r\nAV,521,1,3\r\nAV,521,1,3\r\nAV,521,1,3\r\nAV,521,1,3\r\nAV,521,1,3\r\nAV,521,1,3\r\nAV,521,1,3\r\nAV,521,1,3\r\nAV,521,1,3\r\nAV,521,1,3\r\nAV,521,1,3\r\nAV,521,1,3\r\nAV,521,1,3\r\nAV,521,1,3\r\nAV,521,1,3\r\nAV,521,1,3\r\nAV,521,1,3\r\nAV,521,1,3\r\nAV,521,1,3\r\nAV,521,1,3\r\nAV,521,1,3\r\nAV,521,1,3\r\nAV,521,1,3\r\nAV,521,1,3\r\nAV,521,1,3\r\nAV,521,1,3\r\nAV,521,1,3\r\nAV,521,1,3\r\nAV,521,1,3\r\nAV,521,1,3\r\nAV,521,1,3\r\nAV,521,1,3\r\nAV,521,1,3\r\nAV,521,1,3\r\nAV,521,1,3\r\nAV,521,1,3\r\nAV,521,1,3\r\nAV,521,1,3\r\nAV,521,1,3\r\nAV,521,1,3\r\nAV,521,1,3\r\nAV,521,1,3\r\nAV,521,1,3\r\nAV,521,1,3\r\nAV,521,1,3\r\nAV,521,1,3\r\nAV,521,1,3\r\nAV,521,1,3\r\nAV,521,1,3\r\nAV,521,1,3\r\nAV,521,1,3\r\nAV,521,1,3\r\nAV,521,1,3\r\nAV,521,1,3\r\nAV,521,1,3\r\nAV,521,1,3\r\nAV,521,1,3\r\nAV,521,1,3\r\nAV,521,1,3\r\nAV,521,1,3\r\nAV,521,1,3\r\nAV,521,1,3\r\nAV,521,1,3\r\nAV,521,1,3\r\nAV,521,1,3\r\nAV,521,1,3\r\nAV,521,1,3\r\nAV,521,1,3\r\nAV,521,1,3\r\nAV,521,1,3\r\nAV,521,1,3\r\nAV,521,1,3\r\nAV,521,1,3\r\nAV,521,1,3\r\nAV,521,1,3\r\nAV,521,1,3\r\nAV,521,1,3\r\nAV,521,1,3\r\nAV,521,1,3\r\nAV,521,1,3\r\nAV,521,1,3\r\nAV,521,1,3\r\nAV,521,1,3\r\nAV,521,1,3\r\nAV,521,1,3\r\nAV,521,1,3\r\nAV,521,1,3\r\nAV,521,1,3\r\nAV,521,1,3\r\nAV,521,1,3\r\nAV,521,1,3\r\nAV,521,1,3\r\nAV,521,1,3\r\nAV,521,1,3\r\nAV,521,1,3\r\nAV,521,1,3\r\nAV,521,1,3\r\nAV,521,1,3\r\nAV,521,1,3\r\n"
  out "size(s)":i32[](array[numeric])
  out "AO SampClk.Rate":dbl
  out "Datapoints":i32
  out "Aout Frequency":dbl
  out "Script":T3(array[cluster])=[{"Delay 10µs"=0, "command"=218103809, "P0"=255, "P1"=7, "P2"=0, "P3"=0, "P4"=0, "P5-ticket"=0}, {"Delay 10µs"=0, "command"=4060086273, "P0"=1, "P1"=10, "P2"=0, "P3"=0, "P4"=0, "P5-ticket"=0}, {"Delay 10µs"=50000, "command"=218103809, "P0"=255, "P1"=1, "P2"=0, "P3"=0, "P4"=0, "P5-ticket"=0}, {"Delay 10µs"=50000, "command"=100663297, "P0"=2048, "P1"=131072, "P2"=0, "P3"=0, "P4"=0, "P5-ticket"=0}, {"Delay 10µs"=0, "command"=4043375201, "P0"=-2, "P1"=1, "P2"=0, "P3"=0, "P4"=0, "P5-ticket"=0}, {"Delay 10µs"=0, "command"=4027514895, "P0"=0, "P1"=0, "P2"=0, "P3"=0, "P4"=0, "P5-ticket"=0}] {"command" format="%x" items=["read_x-Motor_status_ticket"=17305600, "init_x-Motor"=17760263, "read_x-Motor_absolute_ticket"=16781312, "move_x-Motor_absolute"=16777217, "move_x-Motor_relative"=16842753, "read_y-Motor_status_ticket"=18354176, "init_y-Motor"=18808839, "read_y-Motor_absolute_ticket"=17829888, "move_y-Motor_absolute"=17825793, "move_y-Motor_relative"=17891329, "read_z-Motor_status_ticket"=19402752, "init_z-Motor"=19857415, "stop_z-Motor"=19857423, "start_z-Motor"=19857422, "read_z-Motor_absolute_ticket"=18878464, "move_z-Motor_absolute"=18874369, "move_z-Motor_relative"=18939905, "end_no_ticket"=4027514895, "end_ticket"=4027518991, "IO-read_bank0"=3489665024, "IO-write_bank0"=3489660929, "IO-read_bank1"=3506442240, "IO-write_bank1"=3506438145, "Analog-write_DA0-0"=2684354561, "Analog-write_DA0-1"=2685403137, "Analog-write_DA0-2"=2686451713, "Analog-write_DA0-3"=2687500289, "Analog-write_DA0-4"=2688548865, "Analog-write_DA0-5"=2689597441, "Analog-write_DA0-6"=2690646017, "Analog-write_DA0-7"=2691694593, "Analog-write_DA1-0"=2701131777, "Analog-write_DA1-1"=2702180353, "Analog-write_DA1-2"=2703228929, "Analog-write_DA1-3"=2704277505, "Analog-write_DA1-4"=2705326081, "Analog-write_DA1-5"=2706374657, "Analog-write_DA1-6"=2707423233, "Analog-write_DA1-7"=2708471809, "Analog-read_AD0-0"=2818576384, "Analog-read-store_AD0-0"=2818572290, "IO-delay_bank0"=3489923073, "IO-delay_bank0_fromVar"=3489923075, "read_cam_clock"=3289124864, "store_cam_clock"=3289120770, "read_cam_phase"=3289190400, "set_cam_deadtime"=3288989697, "set_cam_10uscycles"=3289055233, "set_cam_10uscycles_fromVariable"=3289055235, "calc_cam"=3289317386, "store_cam_Var"=3289251842, "math_addToVariable"=4060086278, "readVar"=4060090368, "writeVar"=4060086273, "copyVar"=4060086276, "decrement_branchRel_if_equal"=4043374945, "decrement_branchRel_if_greaterequal"=4043375201, "decrement_branchRel_if_greaterequal_withTicket"=4043379297, "decrement_branchRel_if_smaller"=4043375457, "increment_branchRel_if_smaller"=4043375473, "set_x-Galvo"=1612710129, "set_y-Galvo"=1613758705, "set_z-Fokus"=1614807281, "set_x-Galvo_position-only"=1612709953, "set_y-Galvo_position-only"=1613758529, "set_z-Fokus_position-only"=1614807105, "set_x-Galvo_position-only_ticket"=1612714049, "set_y-Galvo_position-only_ticket"=1613762625, "set_z-Fokus_position-only_ticket"=1614811201, "set_x-Galvo_speed-only"=1612709921, "set_y-Galvo_speed-only"=1613758497, "set_z-Fokus_speed-only"=1614807073, "read_x-Galvo_ticket"=1612714048, "read_y-Galvo_ticket"=1613762624, "read_z-Focus_ticket"=1614811200, "x-Galvo_pos_fromVar"=1612709955, "y-Galvo_pos_fromVar"=1613758531, "z-Focus_pos_fromVar"=1614807107]; "P0" format="%x"}
  out "siam-commands":i32
  # "Connect PFI6 with PFI0/AI Start"
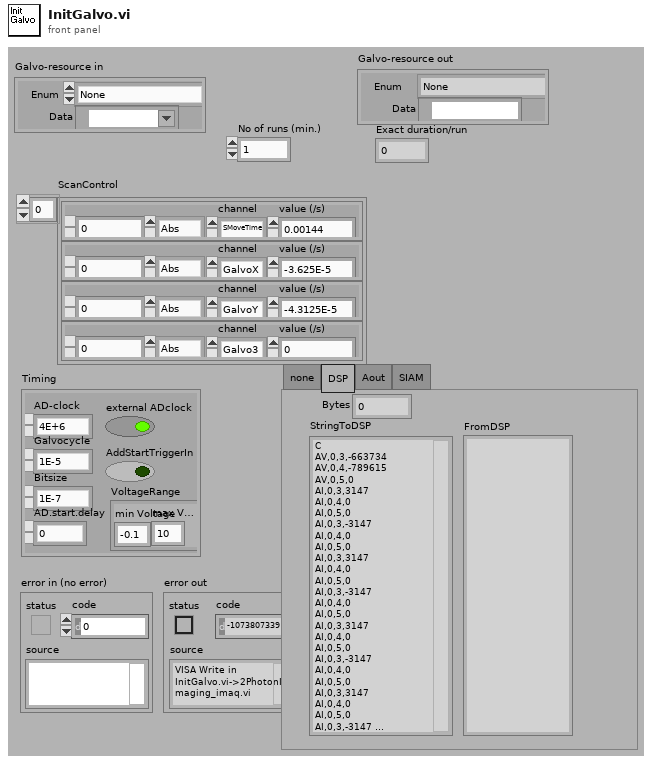
[diagram p1: front panel]
types:
  T1 = cluster{"AD-clock":dbl, "external ADclock":bool, "Galvocycle":dbl, "Bitsize":dbl, "AD.start.delay":dbl, "AddStartTriggerIn":bool, "VoltageRange":cluster{"min Voltage":dbl, "max Voltage":dbl}}
  T2 = typedef "SIAM_command.ctl" = u32
  T3 = cluster{"Delay 10µs":u32, "command":T2, "P0":i32, "P1":i32, "P2":i32, "P3":i32, "P4":i32, "P5-ticket":i32}[]
  T4 = cluster{"Enum":enum16{"None", "DSP-on serial port", "Analog out", "SIAM-withDSiam"}, "Data":refnum<k21>}
  T5 = typedef "ScanControl.ctl" = cluster{"Time [s]":dbl, "action":T6, "channel":T7, "value (/s)":dbl}[]
  T6 = typedef "ScanControl_Action.ctl" = enum16{"Abs", "Rel", "Inc", "IncInc", "LoopStart", "LoopEnd", "WaitTriggerRising"}
  T7 = typedef "ScanControl_Channel.ctl" = enum16{"Com", "AnalogConfig", "AnalogValue", "GalvoX", "GalvoY", "Galvo3", "Galvo4", "Digital", "Free", "Loop", "SMoveTime", "Image1X", "Image1Y", "Image2X", "Image2Y"}
  T8 = enum16{"None", "DSP-on serial port", "Analog out"}
  T9 = enum16{"None", "DSP-on serial port", "Analog out", "SIAM-withDSiam"}
  T10 = typedef "SIAM-send.ctl" = enum16{"validID", "storeID", "enable", "rundirect", "sendlist", "run", "stop", "readRegister", "sendValue", "storeStatus"}
  T11 = enum16{"Com", "AnalogConfig", "AnalogValue", "GalvoX", "GalvoY", "Galvo3", "Galvo4", "Digital", "Free", "Loop", "SMoveTime", "Image1X", "Image1Y", "Image2X", "Image2Y"}[]
  T12 = cluster{"Time [s]":dbl, "action":T6, "channel":T7, "value (/s)":dbl}
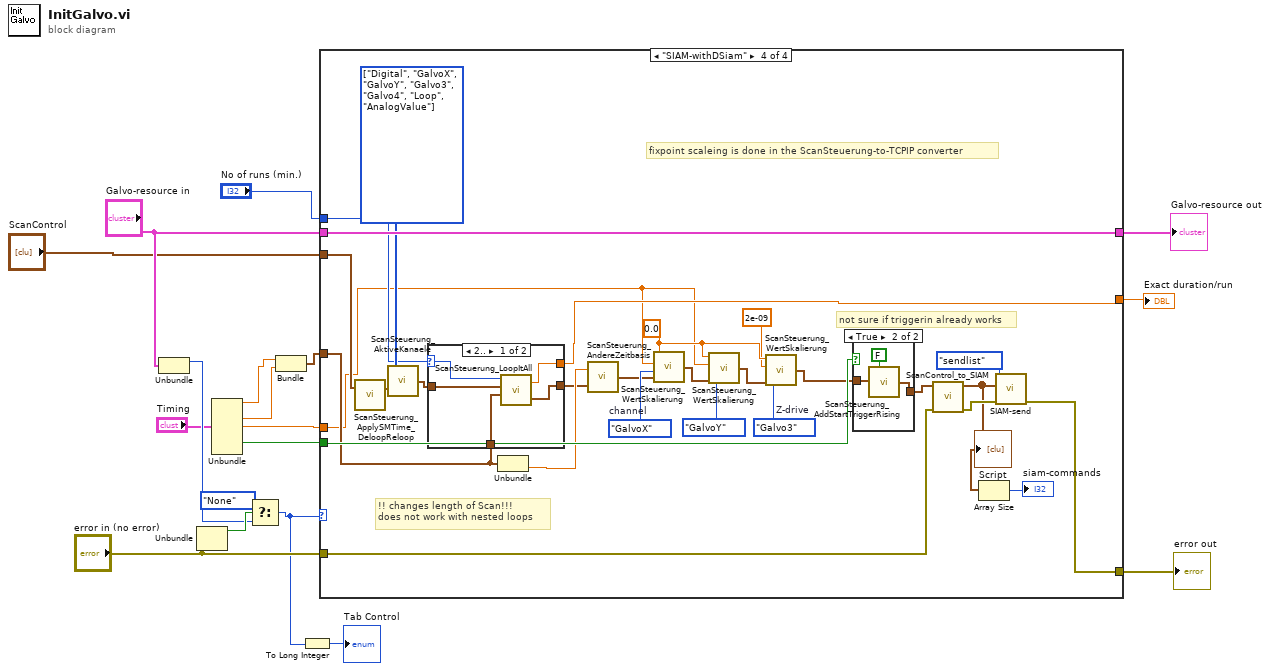
[diagram p0: block diagram]
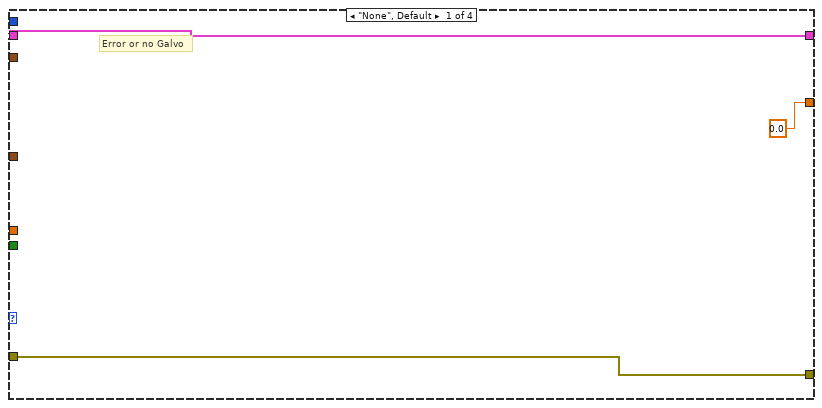
[diagram p2: hidden frame]
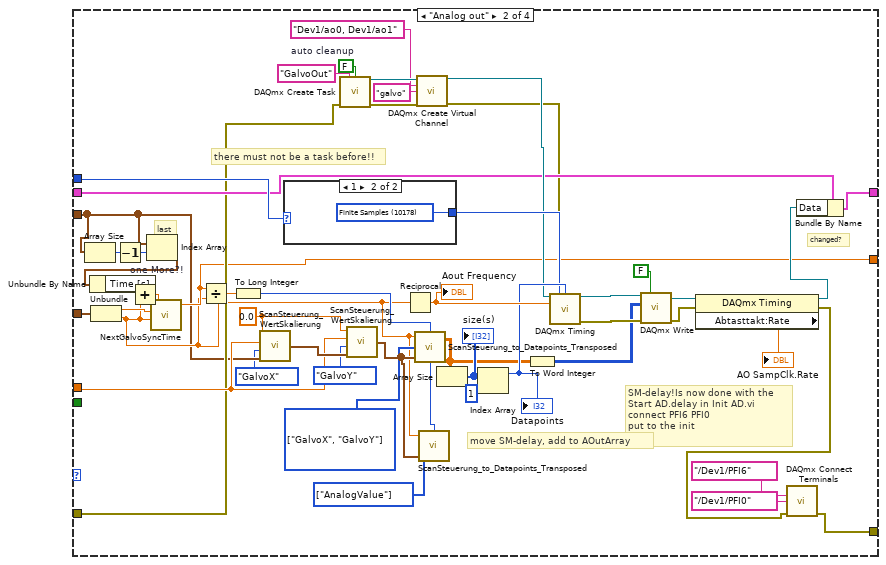
[diagram p3: hidden frame]
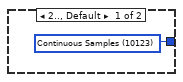
[diagram p4: hidden frame]
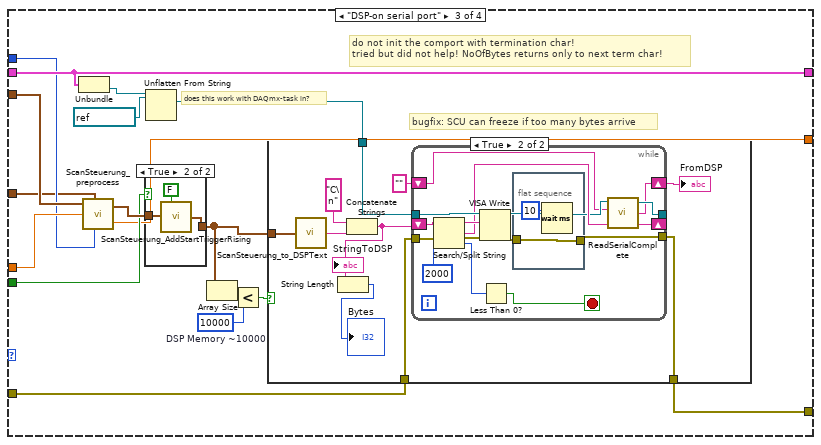
[diagram p5: hidden frame]
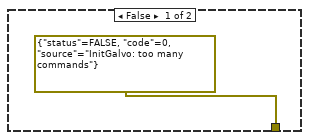
[diagram p6: hidden frame]
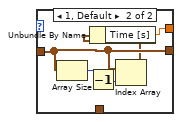
[diagram p8: hidden frame]
diagram:
  n1 = Unbundle("Galvo-resource in") -> ("Enum"=w15:T9)  [unwired: 1 out]
  n2 = Unbundle("error in (no error)") -> ("status"=w16:bool)  [unwired: 2 out]
  n3 = Unbundle("Timing") -> ("AD-clock"=w4:dbl, "Galvocycle"=w3:dbl, "Bitsize"=w1:dbl, "AddStartTriggerIn"=w5:bool)  [unwired: 3 out]
  n4 = Select(t=T8."None", s=w16, f=w15) -> (s? t:f=w11:T9)
  n5 = Bundle("AD-clock"=w4, "Galvocycle"=w3) -> (w2:cluster{"AD-clock":dbl, "Galvocycle":dbl})  [unwired: 1 out]
  n6 = To Long Integer(number=w11) -> (32bit integer=→"Tab Control":i32)
  n7 = case shown="\"SIAM-withDSiam\"" w11 {
    tunnel: "error in (no error)" -> [w21 w42 w90 w145]
    tunnel: [w21 w24 w82 w143] -> w18
    tunnel: "Galvo-resource in" -> [w20 w45 w87 w149]
    tunnel: [w20 w52 w87 w149] -> w12
    tunnel: "ScanControl" -> [_ w30 w84 w135]
    tunnel: w1 -> [_ w61 w85 w123]
    tunnel: "No of runs (min.)" -> [_ w60 w83 w132]
    tunnel: [0.0 ("next GalvoSyncTime") w37 w78 w133] -> w6
    tunnel: w5 -> [_ _ w80 w148]
    tunnel: w2 -> [_ w36 w79 w134]
    frame "None", Default {
      # "Error or no Galvo"
    }
    frame "Analog out" {
      w38 = T11 [enum."AnalogValue"] items=["Com", "AnalogConfig", "AnalogValue", "GalvoX", "GalvoY", "Galvo3", "Galvo4", "Digital", "Free", "Loop", "SMoveTime", "Image1X", "Image1Y", "Image2X", "Image2Y"] ("Aktiv")
      w57 = T11 [enum."GalvoX", enum."GalvoY"] items=["Com", "AnalogConfig", "AnalogValue", "GalvoX", "GalvoY", "Galvo3", "Galvo4", "Digital", "Free", "Loop", "SMoveTime", "Image1X", "Image1Y", "Image2X", "Image2Y"] ("Aktiv")
      w69 = 0.0
      w51 = FALSE  # auto cleanup
      # "last"
      # "move SM-delay, add to AOutArray"
      # "there must not be a task before!!"
      # "changed?"
      # "SM-delay!Is now done with the\nStart AD.delay in Init AD.vi\nconnect PFI6 PFI0\nput to the init"
      n8 = Array Size(array=w30) -> (size(s)=w31:i32)
      n9 = Unbundle(w36) -> ("AD-clock"=w35:dbl, "Galvocycle"=w34:dbl)
      n10 = Decrement(x=w31) -> (x-1=w29:i32)
      n11 = Index Array(array=w30, index=w29) -> (element=w32:T12)
      n12 = Unbundle By Name(w32) -> ("Time [s]"=w28:dbl)
      n13 = Add "one More?!"(x=w28, y=w34) -> (x+y=w33:dbl)
      n14 = call "NextGalvoSyncTime.vi"("Galvocycle [s]"=w34, "AD-Frquency [Hz]"=w35, "Timepoint"=w33) -> ("next GalvoSyncTime"=w37:dbl)  [unwired: 1 in, 2 out]
      n15 = Divide(x=w37, y=w34) -> (x/y=w58:dbl)
      n16 = To Long Integer(number=w58) -> (32bit integer=w40:i32)
      n17 = call "ScanSteuerung_WertSkalierung.vi"("ScanSteuerung"=w30, "Channel"=ScanControl_Channel."GalvoX", "/Skalierung (m/bit)"=w61, "+Offset (m)"=w69) -> ("ScanSteuerungOut"=w68:T5)
      n18 = case shown="1" w60 {
        tunnel: [w72 w73] -> w59
        frame 2.., Default {
          w72 = 10123 items=["Finite Samples"=10178, "Continuous Samples"=10123, "Hardware Timed Single Point"=12522] ("sample mode")
        }
        frame 1 {
          w73 = 10178 items=["Finite Samples"=10178, "Continuous Samples"=10123, "Hardware Timed Single Point"=12522] ("sample mode")
        }
      }
      n19 = call <vilib>:"DAQmx Create Task.vi"("new task name"="GalvoOut", "auto cleanup"=w51, "error in"=w42) -> ("task out"=w50:refnum<k21>, "error out"=w49:errorcluster)  [unwired: 2 in, 9 out]
      n20 = call "ScanSteuerung_WertSkalierung.vi"("ScanSteuerung"=w68, "Channel"=ScanControl_Channel."GalvoY", "/Skalierung (m/bit)"=w61, "+Offset (m)"=w69) -> ("ScanSteuerungOut"=w39:T5)
      n21 = Reciprocal(x=w34) -> (1/x=w67:dbl)
      "Aout Frequency" <- w67
      n22 = call "ScanSteuerung_to_Datapoints_Transposed.vi"("Datapoints (-1=estimate)"=w40, "ScanSteuerung"=w39, "Aktiv"=w57, "Neues Zeitraster"=w34) -> ("Waveform Graph"=w56:dbl[][])  [unwired: 1 out]
      n23 = call-poly <vilib>:"DAQmx Create Virtual Channel.vi"("task in"=w50, "physical channels"="Dev1/ao0, Dev1/ao1" ("names out"), "name to assign"="galvo", "error in"=w49) -> ("task out"=w46:refnum<k21>, "error out"=w44:errorcluster)  [unwired: 5 in, 5 out]
      n24 = call "ScanSteuerung_to_Datapoints_Transposed.vi"("Datapoints (-1=estimate)"=w40, "ScanSteuerung"=w39, "Aktiv"=w38, "Neues Zeitraster"=w34) -> ()  [unwired: 2 out]
      n25 = Array Size(array=w56) -> (size(s)=w70:i32[])
      "size(s)" <- w70
      n26 = Index Array(array=w70, index=1) -> (element=w66:i32)
      "Datapoints" <- w66
      n27 = To Word Integer(number=w56) -> (16bit integer=w41:i16[][])
      n28 = call-poly <vilib>:"DAQmx Timing.vi"("task/channels in"=w46, "sample mode"=w59, "samples per channel"=w66, "rate"=w67, "error in"=w44) -> ("task out"=w54:refnum<k21>, "error out"=w55:errorcluster)  [unwired: 2 in, 7 out]
      n29 = call-poly <vilib>:"DAQmx Write.vi"("task/channels in"=w54, "auto start"=FALSE, "data"=w41, "error in"=w55) -> ("task out"=w64:refnum<k21>, "error out"=w62:errorcluster)  [unwired: 10 out]
      n30 = property class="DAQmx Timing"(reference=w64, error in=w62) -> (reference out=w53:refnum<k21>, error out=w25:errorcluster, "Abtasttakt:Rate"=→"AO SampClk.Rate":dbl)
      n31 = call <vilib>:"DAQmx Connect Terminals.vi"("source terminal"=tag "/Dev1/PFI6", "destination terminal"=tag "/Dev1/PFI0", "error in"=w25) -> ("error out"=w24:errorcluster)  [unwired: 1 in, 11 out]
      n32 = Bundle By Name(cluster=w45, "Data"=w53) -> (w52:T4)
    }
    frame "DSP-on serial port" {
      w75 = 10000  # DSP Memory ~10000
      # "bugfix: SCU can freeze if too many bytes arrive"
      # "does this work with DAQmx-task in?"
      # "do not init the comport with termination char!\ntried but did not help! NoOfBytes returns only to next term char!"
      n33 = Unbundle(w87) -> ("Data"=w89:refnum<k21>)  [unwired: 1 out]
      n34 = call "ScanSteuerung_preprocess.vi"("ScanSteuerung"=w84, "needed constants"=w79, "Skalierung (m/bit)"=w85, "No of loops (min.)"=w83) -> ("ScanSteuerungOut"=w81:T5, "Looptime (1 image)"=w78:dbl)  [unwired: 1 in]
      n35 = case shown="True" w80 {
        tunnel: w81 -> [w118 w121]
        tunnel: [w118 w120] -> w77
        frame False {
        }
        frame True {
          n36 = call "ScanSteuerung_AddStartTriggerRising.vi"("ScanSteuerung 2"=w121, "Care for SmartMove"=FALSE) -> ("ScanSteuerung"=w120:T5)
        }
      }
      n37 = Unflatten From String(type=refnum<visa-resource-name> "COM1" ("DSP resource name"), binary string=w89) -> (value=w86:refnum<visa-resource-name>)  [unwired: 1 in, 4 out]
      n38 = Array Size(array=w77) -> (size(s)=w76:i32)
      n39 = Less?(x=w76, y=w75) -> (x < y?=w74:bool)
      n40 = case shown="True" w74 {
        tunnel: w90 -> [_ w100]
        tunnel: w86 -> [_ w99]
        tunnel: [errorcluster {"status"=FALSE, "code"=0, "source"="InitGalvo: too many commands"} ("error out") w96] -> w82
        tunnel: w77 -> [_ w92]
        frame False {
        }
        frame True {
          n41 = call "ScanSteuerung_to_DSPText.vi"("ScanSteuerungOut"=w92) -> ("String"=w95:string)
          n42 = Concatenate Strings("C\n", w95) -> (w98:string)
          "StringToDSP" <- w98
          n43 = String Length(string=w98) -> (length=→"Bytes":i32)
          n44 = while {
            tunnel: w100 -> [w115]
            tunnel: w99 -> [w113]
            tunnel: [w104] -> _
            tunnel: [w112] -> w96
            shift-right: [w109] -> _
            shift-left: w98 -> [w111]
            shift-right: [w103] -> w93
            shift-left: "" ("read buffer") -> [w102]
            stop <- w106 stop-if-true
            n45 = Search/Split String(string=w111, offset (0)=2000) -> (substring before match=w110:string, match + rest of string=w109:string, offset of match=w107:i32)  [unwired: 1 out]
            n46 = VISA Write(VISA resource name=w113, write buffer=w110, error in (no error)=w115) -> (VISA resource name out=w105:refnum<visa-resource-name>, error out=w114:errorcluster)  [unwired: 1 out]
            n47 = Less Than 0?(x=w107) -> (x < 0?=w106:bool)
            n48 = flat-sequence {
              tunnel: w114 -> [w117]
              tunnel: [w117] -> w112
              frame #0 {
                n49 = Wait (ms)(milliseconds to wait=u32 10) -> ()  [unwired: 1 out]
              }
            }
            n50 = call "ReadSerialComplete.vi"("StringIn"=w102, "duplicate VISA resource name"=w105) -> ("read buffer"=w103:string, "duplicate VISA resource name 2"=w104:refnum<visa-resource-name>)  [unwired: 2 in, 1 out]
          }
          "FromDSP" <- w93
        }
      }
    }
    frame "SIAM-withDSiam" {
      w125 = ScanControl_Channel."Galvo3"  # Z-drive
      w131 = ScanControl_Channel."GalvoX"  # channel
      w124 = 0.0
      w139 = T11 [enum."Digital", enum."GalvoX", enum."GalvoY", enum."Galvo3", enum."Galvo4", enum."Loop", enum."AnalogValue"] items=["Com", "AnalogConfig", "AnalogValue", "GalvoX", "GalvoY", "Galvo3", "Galvo4", "Digital", "Free", "Loop", "SMoveTime", "Image1X", "Image1Y", "Image2X", "Image2Y"] ("Aktiv")
      # "fixpoint scaleing is done in the ScanSteuerung-to-TCPIP converter"
      # "!! changes length of Scan!!!\ndoes not work with nested loops"
      # "not sure if triggerin already works"
      n51 = call "ScanSteuerung_ApplySMTime_DeloopReloop.vi"("ScanSteuerung"=w135) -> ("ScanSteuerungOut"=w136:T5)  [unwired: 1 in, 1 out]
      n52 = call "ScanSteuerung_AktiveKanaele.vi"("ScanSteuerung"=w136, "Aktiv"=w139) -> ("ScanSteuerungOut"=w137:T5)
      n53 = case shown="2.." w132 {
        selector: w132 -> [w152 _]
        tunnel: w137 -> [w154 w158]
        tunnel: [w153 w158] -> w138
        tunnel: [w151 w155] -> w133
        tunnel: w134 -> [w150 _]
        frame 2.. {
          n54 = call "ScanSteuerung_LoopItAll.vi"("needed constants"=w150, "ScanSteuerung"=w154, "Times"=w152) -> ("ScanSteuerungOut"=w153:T5, "Looptime (1 image)"=w151:dbl)  [unwired: 1 in]
        }
        frame 1, Default {
          n55 = Array Size(array=w158) -> (size(s)=w159:i32)
          n56 = Decrement(x=w159) -> (x-1=w157:i32)
          n57 = Index Array(array=w158, index=w157) -> (element=w156:T12)
          n58 = Unbundle By Name(w156) -> ("Time [s]"=w155:dbl)
        }
      }
      n59 = Unbundle(w134) -> ("Galvocycle"=w140:dbl)  [unwired: 1 out]
      n60 = call "ScanSteuerung_AndereZeitbasis.vi"("ScanSteuerung"=w138, "Neues Zeitraster"=w140) -> ("ScanSteuerungOut"=w130:T5)
      n61 = call "ScanSteuerung_WertSkalierung.vi"("ScanSteuerung"=w130, "Channel"=w131, "/Skalierung (m/bit)"=w123, "+Offset (m)"=w124) -> ("ScanSteuerungOut"=w129:T5)
      n62 = call "ScanSteuerung_WertSkalierung.vi"("ScanSteuerung"=w129, "Channel"=ScanControl_Channel."GalvoY", "/Skalierung (m/bit)"=w123, "+Offset (m)"=w124) -> ("ScanSteuerungOut"=w128:T5)
      n63 = call "ScanSteuerung_WertSkalierung.vi"("ScanSteuerung"=w128, "Channel"=w125, "/Skalierung (m/bit)"=2e-09, "+Offset (m)"=w124) -> ("ScanSteuerungOut"=w127:T5)
      n64 = case shown="True" w148 {
        tunnel: w127 -> [w160 w163]
        tunnel: [w160 w162] -> w147
        frame False {
        }
        frame True {
          n65 = call "ScanSteuerung_AddStartTriggerRising.vi"("ScanSteuerung 2"=w163, "Care for SmartMove"=FALSE) -> ("ScanSteuerung"=w162:T5)
        }
      }
      n66 = call "ScanControl_to_SIAM.vi"("error in (no error)"=w145, "ScanSteuerung"=w147) -> ("error out"=w144:errorcluster, "Script"=w142:T3)  [unwired: 7 in, 1 out]
      "Script" <- w142
      n67 = Array Size(array=w142) -> (size(s)=→"siam-commands":i32)
      n68 = call "SIAM-send.vi"("error in (no error)"=w144, "Script"=w142, "command"=SIAM-send."sendlist") -> ("error out"=w143:errorcluster)  [unwired: 7 in, 1 out]
    }
  }
  "error out" <- w18
  "Galvo-resource out" <- w12
  "Exact duration/run" <- w6
